vi "Attocube Main.vi"() -> ()   [LabVIEW 2019]
panel:
  out "last move time":timestamp
  out "axis 1:\nCurrent position [µm/°/m°] 2":dbl(knob) scale=65.0..270.0 scale format="%#_3p"
  out "axis 1:\nCurrent position (°)":dbl format="%.4f"
  in  "set static amplitude\nwhen moving":bool
  in  "static amplitude (mV)":dbl=2.0 min=0.001 max=2.0 format="%#_13g"
  in  "both axes: Output":bool caption="both axes:\nOutput"
  in  "axis 2:\nStop moving":bool
  in  "axis 1:\nStop moving":bool
  in  "Remote mode":bool
  in  "axis 2:\nstop detection":bool
  in  "axis 1:\nstop detection":bool
  in  "axis 2:\nOutput":bool
  in  "axis 1:\ncontrol mode":enum16{"speed", "amplitude", "step size"}(ring)=enum."amplitude"
  in  "axis 2:\ncontrol mode":enum16{"speed", "amplitude", "step size"}(ring)=enum."amplitude"
  in  "axis 1:\nOutput":bool
  out "axis 2:\nStepWidth":i32=38 format="%.0fnm"
  out "axis 1:\nStepWidth":i32 format="%.0fnm"
  out "axis 2:\nspeed (°/s)":i32=31
  out "axis 1:\nspeed (°/s)":i32
  out "axis 2:\nCapacitance":i32=2486 format="%.0fnF"
  out "axis 1:\nCapacitance":i32=2534 format="%.0fnF"
  in  "axis 2:\ncap. measure":bool
  in  "axis 1:\ncap. measure":bool
  out "axis 2:\nCurrent position [µm/°/m°] 2":dbl(knob) scale=5.0..320.0
  in  "axis 2:\nFrequency [Hz]":i32=800 min=0 max=20000 format="%.0fHz"
  in  "axis 1:\nFrequency [Hz]":i32=800 min=0 max=20000 format="%.0fHz"
  in  "axis 2:\nDCLevel [V]":dbl min=0.0 max=140.0 step=0.001 format="%.3f"
  in  "axis 1:\nDCLevel [V]":dbl min=0.0 max=140.0 step=0.001 format="%.3f"
  in  "axis 2:\nAmplitude [V]":dbl=35.0 min=0.0 max=150.0 format="%.3gV"
  in  "axis 1:\nAmplitude [V]":dbl=40.0 min=0.0 max=150.0 format="%.3gV"
  in  "axis 2:\ncontinuous back":bool
  in  "axis 2:\ncontinuous fwd":bool
  in  "axis 1:\ncontinuous back":bool
  in  "axis 1:\ncontinuous fwd":bool
  in  "axis 2:\nsingle step fwd":bool
  in  "axis 2:\nsingle step back":bool
  in  "axis 1:\nsingle step back":bool
  in  "axis 1:\nsingle step fwd":bool
  in  "axis 2:\nsp position °":dbl=78.5 min=5.0 max=320.0 format="%.4g"
  in  "axis 2:\nsp rot count":i32
  in  "axis 1:\nsp rot count":i32
  in  "axis 1:\nsp position °":dbl=167.0 min=65.0 max=270.0 format="%.4g"
  in  "axis 2:\nAbsolute":bool
  in  "axis 2:\nRelative":bool
  in  "axis 1:\nRelative":bool
  in  "axis 1:\nAbsolute":bool
  in  "axis 1: \nTarget GND":bool
  in  "axis 1:\nSingle Circle Mode":bool
  in  "axis 2:\nSingle Circle Mode":bool
  in  "axis 2: \nTarget GND":bool
  out "axis 2:\npositioner status":T1
  out "axis 2:\nCurrent position (°)":dbl format="%.4f"
  out "axis 2:\nrot. count":i32
  out "axis 1:\npositioner status":T1
  out "axis 1:\nrot. count":i32
  out "handle":i32=5
  in  "OK":bool
  # "Axis 1: large axis"
  # "Axis 2: small axis"
  # "Notes: \n\n***Switch controller to ground (output=false) before connecting the rotator and while cooling down/warming up***\n\nAxis 1 (large axis): Position is limited by physical stops to angles from 65° to 270°\n\nAxis 2 (small axis): Encoded positions are limited to angles from 5° to 320°, not physically limited to one rotation.  Keep single circle mode OFF to limit the rotation count to zero and protect the wiring from over-rotating.\n\nStatic Amplitude: Sets the voltage applied to the resitive readout system.  Range: 0.001 V to 2V.  Higher voltages enhace the sensitivity but lower voltages minimize heat dissipation for low temperature applications.\n\nAbsolute: positioner travels from its current position to      the target position.\n\nTarget Ground: positioner will be grounded when the target position is reached.\n\nSingle circle mode: If OFF absolute and relative positioning are only allowed up to a full circle, keeps rot count at zero.\n\nOutput: When checked, the repective axis output is enabled.  Deactivating sets the axis to GND\n\nControl mode: \n     amplitude: individual steps of the piezo are definied by        the amplitude.  Driven in open-loop mode, travel speed and step width may vary\n     speed: feedback enables a constant travel speed by closed-loop control of the amplitude and frequency.  Speed is set by adjusting the amplitude and/or frequency values.\n     step width: Step size in controlled to a constant value.  Amplitude is closed-loop controlled.  Step width is set by adjusting the amplitude"
  # "Automatic Positioning"
  # "Automatic Positioning"
  # "Manual Positioning"
  # "Manual Positioning"
  # "Move Single Step"
  # "Move Single Step"
  # "Move Continuous"
  # "Move Continuous"
  # "Capacitance Measurement"
  # "Capacitance Measurement"
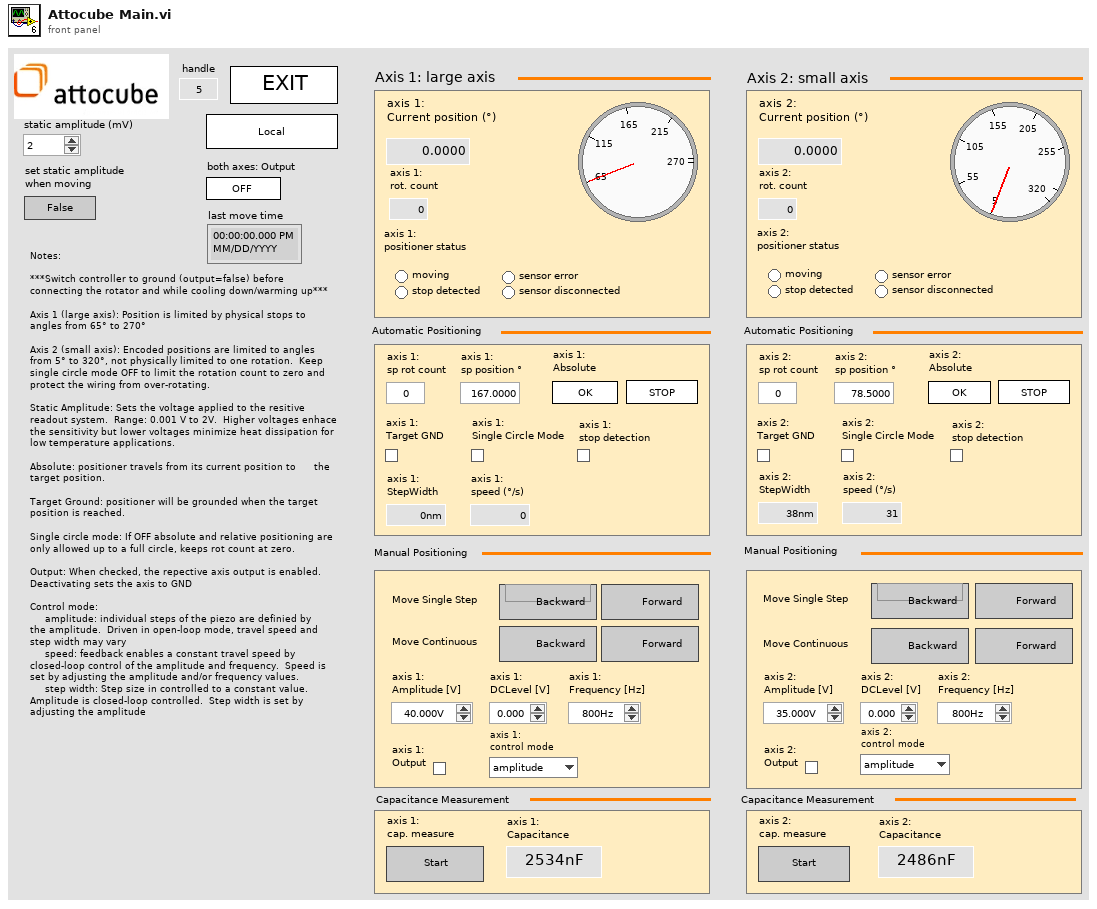
[diagram p1: front panel]
types:
  T1 = cluster{"moving":bool, "stop detected":bool, "sensor error":bool, "sensor disconnected":bool}
  T2 = enum32{"invalid app kind", "Development System", "Run Time System", "Student Edition", "Embedded LabVIEW", "Evaluation", "Custom"}
  T3 = enum32{"Invalid", "Standard", "Closed", "Hidden", "Minimized", "Maximized"}
  T4 = cluster{"axis 1: Absolute":bool, "axis 2: Absolute":bool, "axis 1: Stop moving":bool, "axis 2: Stop moving":bool, "axis 1: Output":bool, "axis 2: Output":bool, "set static amplitude\nwhen moving":bool}
  T5 = cluster{"axis 1: Current position (°)":dbl, "axis 2: Current position (°)":dbl, "axis 1: rot. count":dbl, "axis 2: rot. count":dbl, "axis 1: StepWidth":dbl, "axis 2: StepWidth":dbl, "axis 1: speed (°/s)":dbl, "axis 2: speed (°/s)":dbl, "axis 1: positioner status":cluster{"moving":bool, "stop detected":bool, "sensor error":bool, "sensor disconnected":bool}, "axis 2: positioner status":cluster{"moving":bool, "stop detected":bool, "sensor error":bool, "sensor disconnected":bool}}
  T6 = cluster{"axis 1: Amplitude [V]":dbl, "axis 2: Amplitude [V]":dbl, "axis 1: DCLevel [V]":dbl, "axis 2: DCLevel [V]":dbl, "axis 1: Frequency [Hz]":dbl, "axis 2: Frequency [Hz]":dbl, "axis 1: sp position °":dbl, "axis 2: sp position °":dbl, "axis 1: sp rot count":dbl, "axis 2: sp rot count":dbl}
  T7 = cluster{"error ":bool, "error number":i32, "error code":string}
  T8 = cluster{"Core":cluster{"Current VI Reference":refnum<vi>, "Close Panel on Exit?":bool}, "handle":i32}
  T9 = cluster{"Current VI Reference":refnum<vi>, "Close Panel on Exit?":bool}
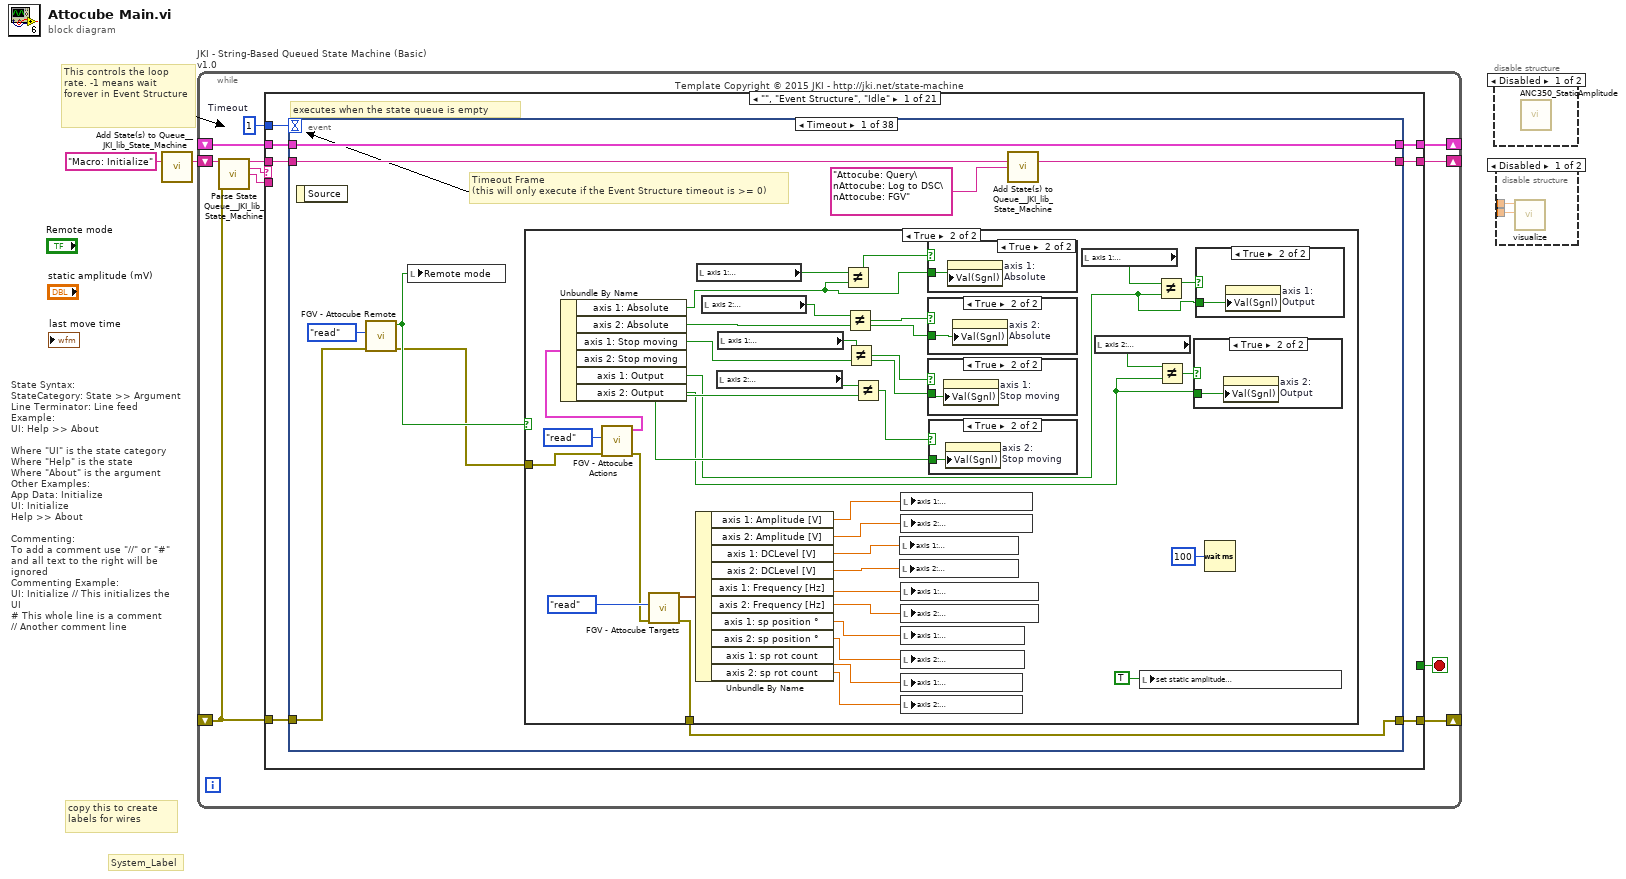
[diagram p0: block diagram]
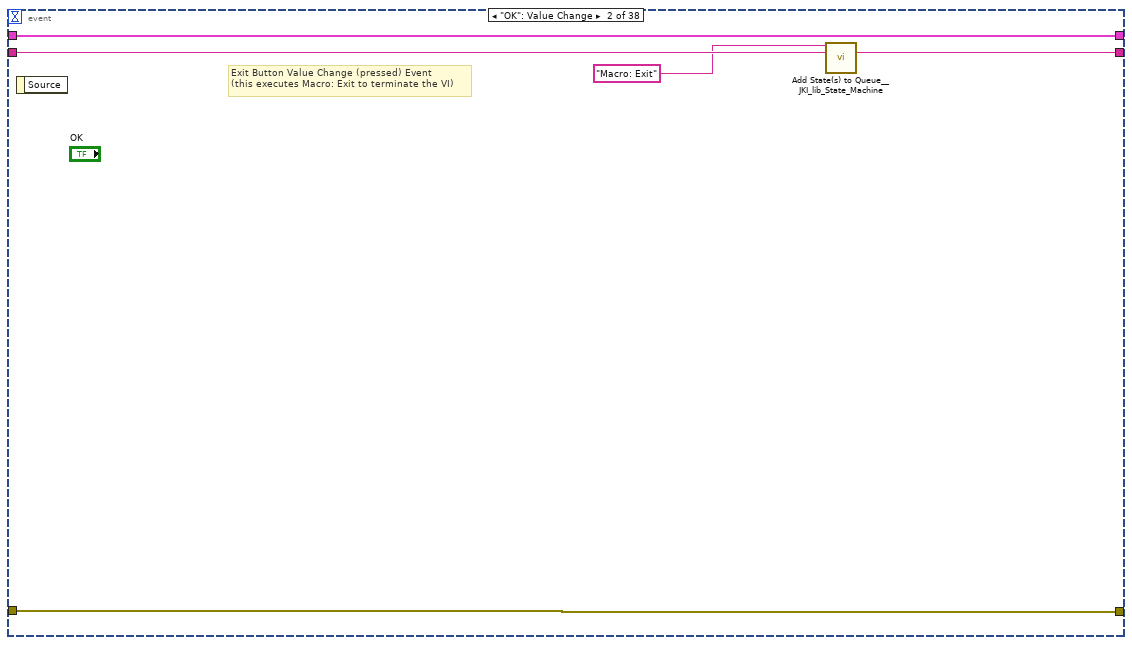
[diagram p11: hidden frame]
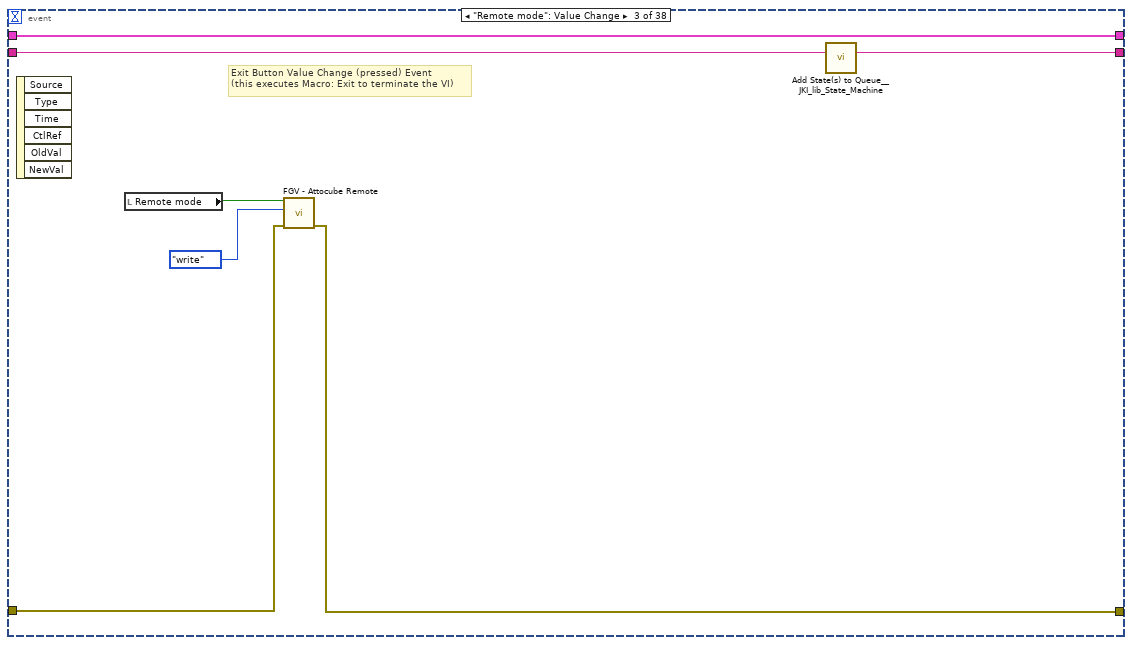
[diagram p12: hidden frame]
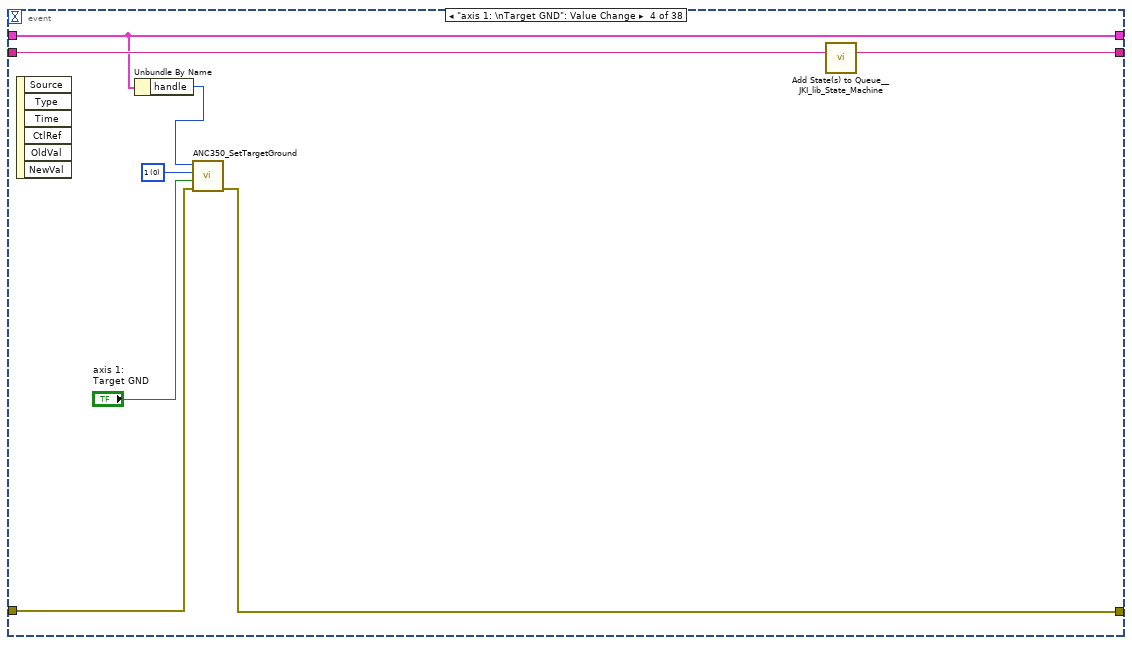
[diagram p13: hidden frame]
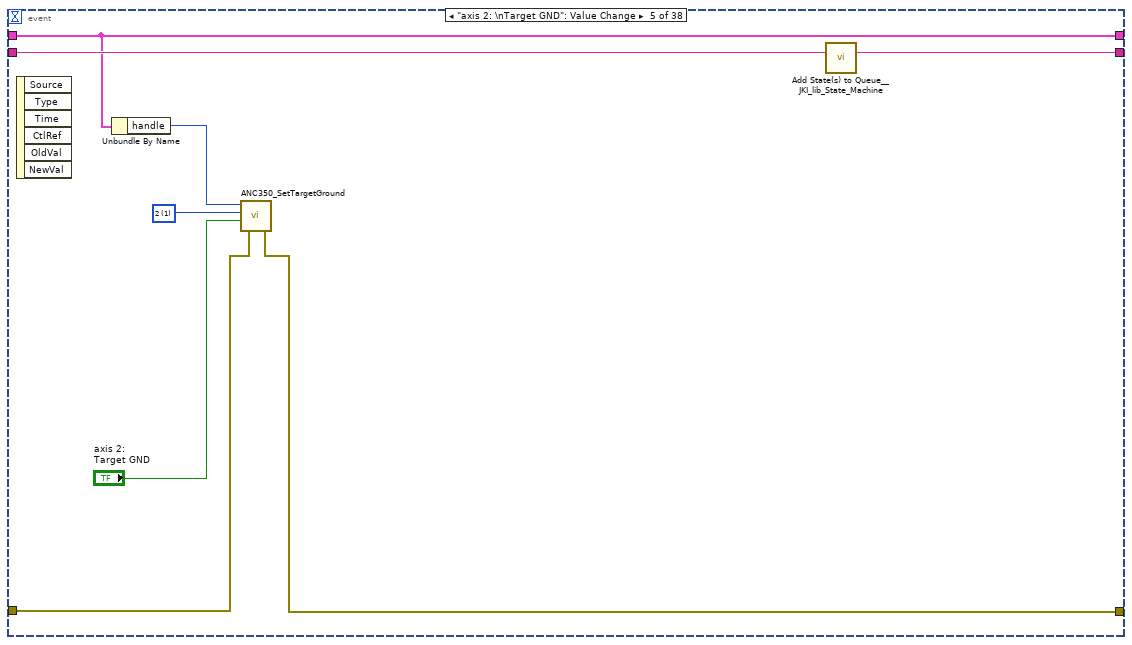
[diagram p14: hidden frame]
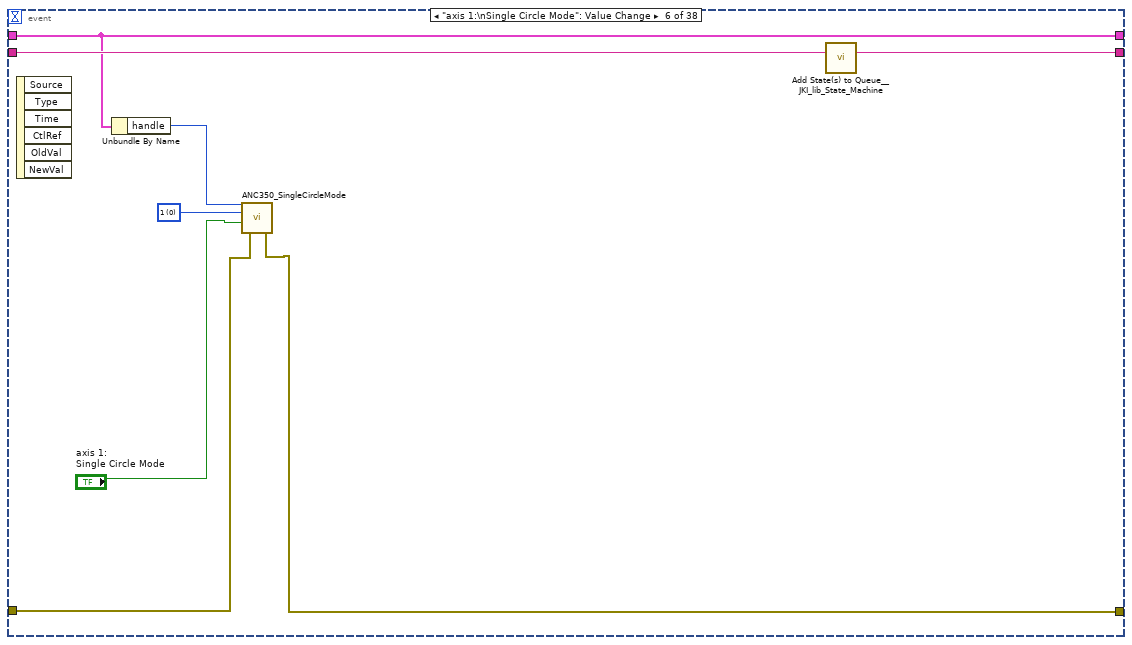
[diagram p15: hidden frame]
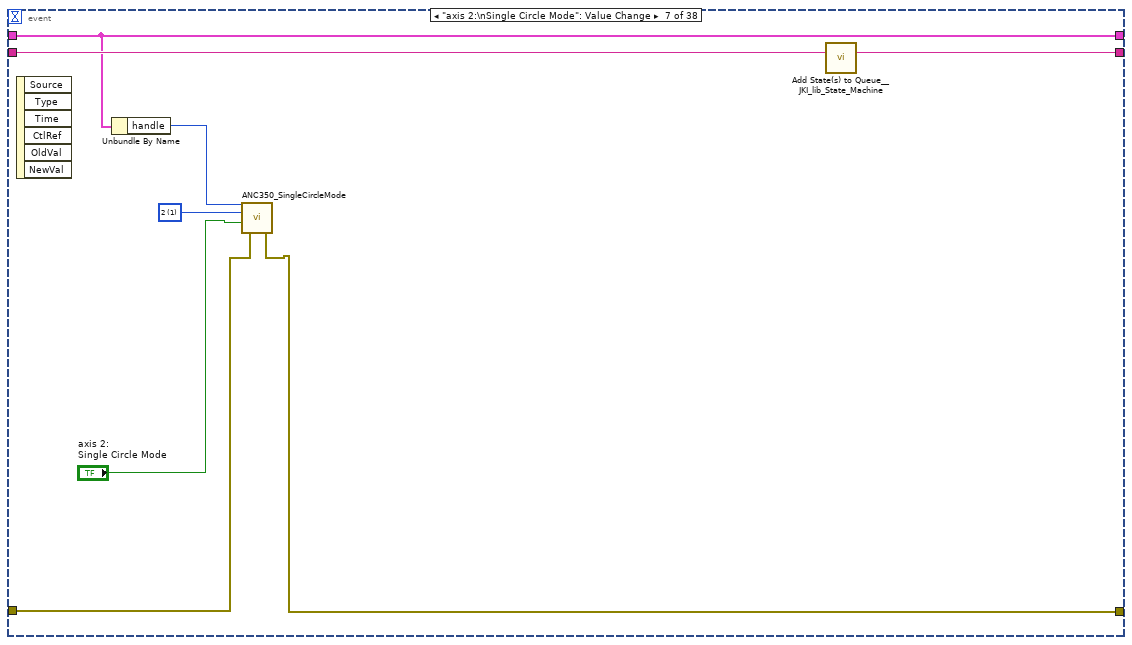
[diagram p16: hidden frame]
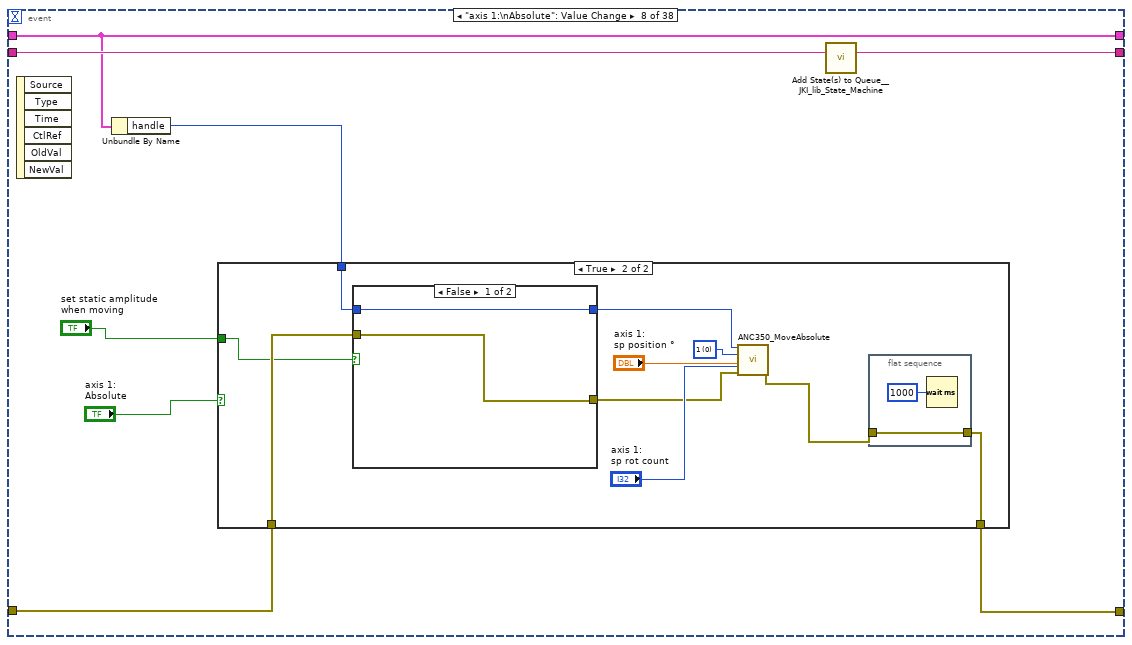
[diagram p17: hidden frame]
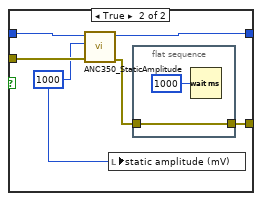
[diagram p19: hidden frame]
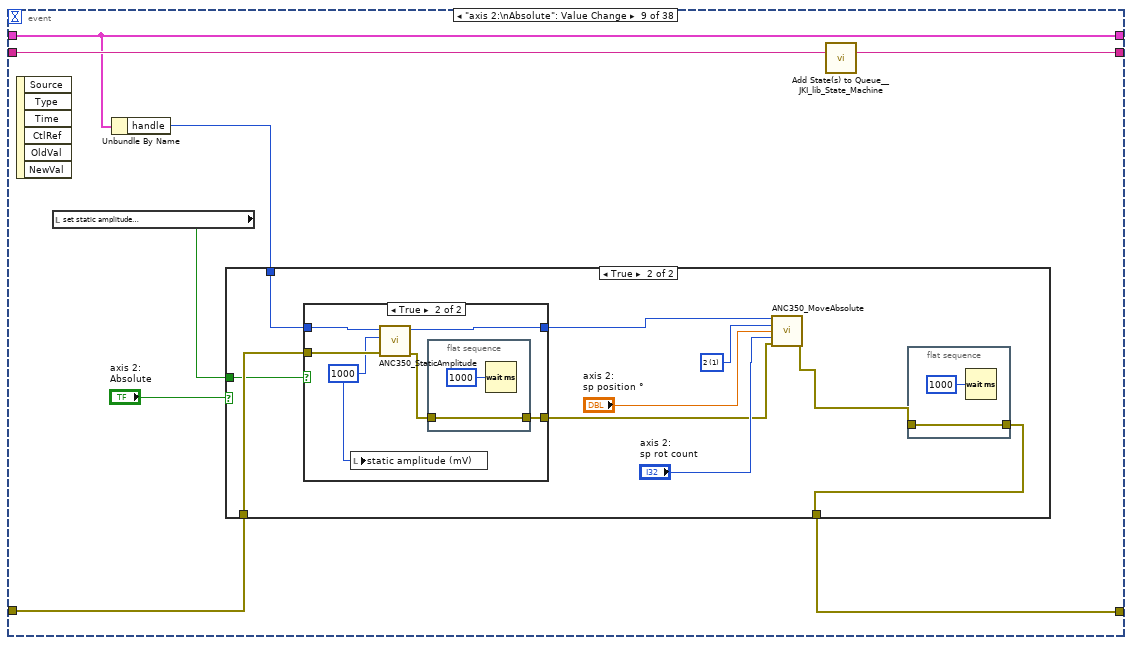
[diagram p20: hidden frame]
diagram:
  # "State Syntax:\nStateCategory: State >> Argument\nLine Terminator: Line feed\nExample:\nUI: Help >> About\n\nWhere \"UI\" is the state category\nWhere \"Help\" is the state\nWhere \"About\" is the argument\nOther Examples:\nApp Data: Initialize\nUI: Initialize\nHelp >> About\n\nCommenting:\nTo add a comment use \"//\" or \"#\" and all text to the right will be ignored\nCommenting Example:\nUI: Initialize // This initializes the UI\n# This whole line is a comment\n// Another comment line"
  # "copy this to create labels for wires"
  # "This controls the loop rate. -1 means wait forever in Event Structure"
  # "System_Label"
  n1 = call <vilib>:"Add State(s) to Queue__JKI_lib_State_Machine.vi"("State(s) in (\"\")"="Macro: Initialize") -> ("States Out"=w2:string)  [unwired: 14 in]
  n2 = while "JKI - String-Based Queued State Machine (Basic) v1.0" {
    shift-right: [w7] -> _
    shift-left: _ -> [w6]
    shift-right: [w3] -> _
    shift-left: _ -> [w4]
    shift-right: [w9] -> _
    shift-left: w2 -> [w10]
    stop <- w8 stop-if-true
    w5 = 1  # Timeout
    # "Template Copyright © 2015 JKI - http://jki.net/state-machine"
    n3 = call <vilib>:"Parse State Queue__JKI_lib_State_Machine.vi"("State Queue"=w10, "Error In (no error)"=w4) -> ("Remaining States"=w12:string, "Current State"=w13:string, "Arguments"=w11:string)  [unwired: 11 in]
    n4 = case shown="\"\", \"Event Structure\", \"Idle\"" w13 {
      selector: w13 -> [_ _ w504 _ _ _ _ _ _ _ _ _ _ _ _ _ _ _ _ _ _]
      tunnel: w12 -> [w20 w503 w508 w526 w532 w537 w541 w547 w553 w557 w568 w579 w590 w616 w621 w647 w651 w666 w736 w797 w850]
      tunnel: w11 -> [_ _ _ _ _ _ _ _ _ _ _ w574 w584 _ _ _ _ _ _ _ _]
      tunnel: w6 -> [w18 w500 w506 w517 w529 w535 w538 _ w548 w554 w566 w577 w586 w613 w618 w645 w648 w664 w734 w795 w848]
      tunnel: w4 -> [w16 w501 w509 w523 w528 w534 w539 w544 w550 w555 w565 w576 w588 w614 w619 w635 w649 _ w733 w750 w815]
      tunnel: [w19 w502 w507 w525 w531 w536 w540 w546 w552 w556 w567 w578 w589 w615 w620 w646 w650 w665 w735 w796 w849] -> w9
      tunnel: [_ _ _ _ _ TRUE _ _ _ _ _ _ _ _ _ _ _ _ _ _ _] -> w8
      tunnel: [w15 w500 w506 w524 w529 w535 w538 w545 w548 w554 w566 w577 w586 w613 w618 w645 w648 w663 w734 w795 w848] -> w7
      tunnel: w5 -> [w14 _ _ _ _ _ _ _ _ _ _ _ _ _ _ _ _ _ _ _ _]
      tunnel: [w17 w501 w510 w523 errorcluster {"status"=FALSE, "code"=0, "source"=""} ("error out") w534 w539 w544 w549 w555 w565 w575 w587 w614 w619 w638 w649 w653 w683 w750 w823] -> w3
      frame "", "Event Structure", "Idle" {
        # "executes when the state queue is empty"
        n5 = event shown="[0] Timeout" {
          selector: _ -> [_ _ _ _ _ _ _ _ _ _ _ _ _ _ _ _ _ _ _ _ _ _ _ _ _ _ _ _ _ _ _ _ _ _ _ _ _ _]
          dyn-events: _ -> [_ _ _ _ _ _ _ _ _ _ _ _ _ _ _ _ _ _ _ _ _ _ _ _ _ _ _ _ _ _ _ _ _ _ _ _ _ _]
          timeout: w14 -> [_ _ _ _ _ _ _ _ _ _ _ _ _ _ _ _ _ _ _ _ _ _ _ _ _ _ _ _ _ _ _ _ _ _ _ _ _ _]
          tunnel: w20 -> [w29 w78 w85 w93 w101 w109 w117 w125 w156 w186 w200 w214 w227 w240 w253 w266 w282 w298 w314 w331 w339 w347 w355 w363 w371 w379 w393 w407 w415 w423 w432 w441 w449 w457 w470 w479 w488 w499]
          tunnel: [w28 w77 w84 w92 w100 w108 w116 w124 w155 w185 w199 w213 w226 w239 w252 w265 w281 w297 w313 w330 w338 w346 w354 w362 w370 w378 w392 w406 w414 w422 w431 w440 w448 w456 w469 w478 w487 w498] -> w19
          tunnel: w18 -> [w27 w75 w83 w91 w99 w107 w115 w123 w154 w184 w198 w212 w225 w238 w251 w264 w280 w296 w312 w329 w337 w345 w353 w361 w369 w377 w391 w405 w413 w421 w430 w439 w447 w455 w468 w477 w486 w496]
          tunnel: [w23 w76 w79 w86 w96 w102 w112 w118 w151 w181 w195 w209 w222 w235 w248 w261 w277 w293 w309 w324 w333 w340 w349 w356 w365 w373 w387 w401 w409 w418 w427 w435 w443 w451 w464 w476 w483 w497] -> w17
          tunnel: w16 -> [w22 w76 w80 w87 w97 w103 w113 w121 w152 w182 w196 w210 w223 w236 w249 w262 w278 w294 w310 w325 w334 w341 w350 w357 w366 w374 w388 w402 w410 w419 w428 w436 w444 w452 w465 w476 w484 w497]
          tunnel: [w27 w75 w83 w91 w99 w107 w115 w123 w154 w184 w198 w212 w225 w238 w251 w264 w280 w296 w312 w329 w337 w345 w353 w361 w369 w377 w391 w405 w413 w421 w430 w439 w447 w455 w468 w477 w486 w496] -> w15
          event Timeout {
            # "Timeout Frame\n(this will only execute if the Event Structure timeout is >= 0)"
            n6 = event-data() -> ()  [unwired: 1 in, 1 out]
            n7 = call "FGV - Attocube Remote.vi"("error in"=w22, "Function"=enum16{"write", "read"}."read") -> ("error out"=w21:errorcluster, "Attocube Remote"=w24:bool)  [unwired: 4 in]
            n8 = local write "Remote mode"(w24) -> ()
            n9 = case shown="True" w24 {
              tunnel: w21 -> [w30 w34]
              tunnel: [w30 w32] -> w23
              frame False {
              }
              frame True {
                n10 = call "FGV - Attocube Actions.vi"("error in"=w34, "Function"=enum16{"write", "read"}."read") -> ("error out"=w33:errorcluster, "Actions OUT"=w66:T4)  [unwired: 4 in]
                n11 = Unbundle By Name(w66) -> ("axis 1: Absolute"=w60:bool, "axis 2: Absolute"=w59:bool, "axis 1: Stop moving"=w55:bool, "axis 2: Stop moving"=w54:bool, "axis 1: Output"=w39:bool, "axis 2: Output"=w36:bool)
                n12 = call "FGV - Attocube Targets.vi"("error in"=w33, "Function"=enum16{"write", "read"}."read") -> ("error out"=w32:errorcluster, "Targets Out"=w52:T6)  [unwired: 4 in]
                n13 = Unbundle By Name(w52) -> ("axis 1: Amplitude [V]"=w51:dbl, "axis 2: Amplitude [V]"=w50:dbl, "axis 1: DCLevel [V]"=w49:dbl, "axis 2: DCLevel [V]"=w48:dbl, "axis 1: Frequency [Hz]"=w47:dbl, "axis 2: Frequency [Hz]"=w46:dbl, "axis 1: sp position °"=w31:dbl, "axis 2: sp position °"=w45:dbl, "axis 1: sp rot count"=w44:dbl, "axis 2: sp rot count"=w43:dbl)
                n14 = local read "axis 1:\nAbsolute"() -> (w65:bool)
                n15 = local read "axis 2:\nAbsolute"() -> (w64:bool)
                n16 = local read "axis 2:\nStop moving"() -> (w62:bool)
                n17 = local read "axis 1:\nStop moving"() -> (w63:bool)
                n18 = Not Equal?(x=w65, y=w60) -> (x != y?=w61:bool)
                n19 = Not Equal?(x=w64, y=w59) -> (x != y?=w58:bool)
                n20 = Not Equal?(x=w63, y=w55) -> (x != y?=w57:bool)
                n21 = Not Equal?(x=w62, y=w54) -> (x != y?=w56:bool)
                n22 = local write "axis 1:\nDCLevel [V]"(w49) -> ()
                n23 = local write "axis 2:\nDCLevel [V]"(w48) -> ()
                n24 = local write "axis 1:\nAmplitude [V]"(w51) -> ()
                n25 = local write "axis 2:\nAmplitude [V]"(w50) -> ()
                n26 = local write "axis 1:\nFrequency [Hz]"(w47) -> ()
                n27 = local write "axis 2:\nFrequency [Hz]"(w46) -> ()
                n28 = local write "axis 1:\nsp position °"(w31) -> ()
                n29 = local write "axis 2:\nsp position °"(w45) -> ()
                n30 = local write "axis 1:\nsp rot count"(w44) -> ()
                n31 = local write "axis 2:\nsp rot count"(w43) -> ()
                n32 = case shown="True" w61 {
                  tunnel: w60 -> [_ w73]
                  frame False {
                  }
                  frame True {
                    n33 = property on="axis 1:\nAbsolute" class="Bool (strict)"("Val(Sgnl)"=w73) -> ()  [unwired: 2 in, 2 out]
                  }
                }
                n34 = case shown="True" w58 {
                  tunnel: w59 -> [_ w72]
                  frame False {
                  }
                  frame True {
                    n35 = property on="axis 2:\nAbsolute" class="Bool (strict)"("Val(Sgnl)"=w72) -> ()  [unwired: 2 in, 2 out]
                  }
                }
                n36 = case shown="True" w57 {
                  tunnel: w55 -> [_ w71]
                  frame False {
                  }
                  frame True {
                    n37 = property on="axis 1:\nStop moving" class="Bool (strict)"("Val(Sgnl)"=w71) -> ()  [unwired: 2 in, 2 out]
                  }
                }
                n38 = case shown="True" w56 {
                  tunnel: w54 -> [_ w70]
                  frame False {
                  }
                  frame True {
                    n39 = property on="axis 2:\nStop moving" class="Bool (strict)"("Val(Sgnl)"=w70) -> ()  [unwired: 2 in, 2 out]
                  }
                }
                n40 = local read "axis 1:\nOutput"() -> (w40:bool)
                n41 = local read "axis 2:\nOutput"() -> (w37:bool)
                n42 = local write "set static amplitude\nwhen moving"(TRUE) -> ()
                n43 = Not Equal?(x=w40, y=w39) -> (x != y?=w41:bool)
                n44 = Not Equal?(x=w37, y=w36) -> (x != y?=w38:bool)
                n45 = case shown="True" w38 {
                  tunnel: w36 -> [_ w68]
                  frame False {
                  }
                  frame True {
                    n46 = property on="axis 2:\nOutput" class="Bool (strict)"("Val(Sgnl)"=w68) -> ()  [unwired: 2 in, 2 out]
                  }
                }
                n47 = case shown="True" w41 {
                  tunnel: w39 -> [_ w69]
                  frame False {
                  }
                  frame True {
                    n48 = property on="axis 1:\nOutput" class="Bool (strict)"("Val(Sgnl)"=w69) -> ()  [unwired: 2 in, 2 out]
                  }
                }
                n49 = Wait (ms)(milliseconds to wait=u32 100) -> ()  [unwired: 1 out]
              }
            }
            n50 = call <vilib>:"Add State(s) to Queue__JKI_lib_State_Machine.vi"("State(s) in (\"\")"=w29, "State(s) at Back (\"\")"="Attocube: Query\nAttocube: Log to DSC\nAttocube: FGV" ("State(s) at Back (\"\")")) -> ("States Out"=w28:string)  [unwired: 13 in]
          }
          event "OK": Value Change {
            # "Exit Button Value Change (pressed) Event\n(this executes Macro: Exit to terminate the VI)"
            n51 = event-data() -> ()  [unwired: 1 in, 1 out]
            n52 = call <vilib>:"Add State(s) to Queue__JKI_lib_State_Machine.vi"("State(s) in Front (\"\")"="Macro: Exit", "State(s) in (\"\")"=w78) -> ("States Out"=w77:string)  [unwired: 13 in]
          }
          event "Remote mode": Value Change {
            # "Exit Button Value Change (pressed) Event\n(this executes Macro: Exit to terminate the VI)"
            n53 = event-data() -> ()  [unwired: 1 in, 6 out]
            n54 = local read "Remote mode"() -> (w82:bool)
            n55 = call "FGV - Attocube Remote.vi"("error in"=w80, "Function"=enum16{"write", "read"}."write", "Attocube Remote"=w82) -> ("error out"=w79:errorcluster)  [unwired: 3 in, 1 out]
            n56 = call <vilib>:"Add State(s) to Queue__JKI_lib_State_Machine.vi"("State(s) in (\"\")"=w85) -> ("States Out"=w84:string)  [unwired: 14 in]
          }
          event "axis 1: \nTarget GND": Value Change {
            w89 = u8 0 items=["1", "2", "3", "4", "5", "6", "7", "8", "9"] ("axis no")
            n57 = event-data() -> ()  [unwired: 1 in, 6 out]
            n58 = Unbundle By Name(w91) -> ("handle"=w90:i32)
            n59 = call "ANC350_SetTargetGround.vi"("error in"=w87, "PositionerAcIn"="axis 1: \nTarget GND", "axis no"=w89, "device handle"=w90) -> ("error out"=w86:T7)  [unwired: 2 in, 1 out]
            n60 = call <vilib>:"Add State(s) to Queue__JKI_lib_State_Machine.vi"("State(s) in (\"\")"=w93) -> ("States Out"=w92:string)  [unwired: 14 in]
          }
          event "axis 2: \nTarget GND": Value Change {
            w95 = u8 1 items=["1", "2", "3", "4", "5", "6", "7", "8", "9"] ("axis no")
            n61 = event-data() -> ()  [unwired: 1 in, 6 out]
            n62 = Unbundle By Name(w99) -> ("handle"=w98:i32)
            n63 = call "ANC350_SetTargetGround.vi"("error in"=w97, "PositionerAcIn"="axis 2: \nTarget GND", "axis no"=w95, "device handle"=w98) -> ("error out"=w96:T7)  [unwired: 2 in, 1 out]
            n64 = call <vilib>:"Add State(s) to Queue__JKI_lib_State_Machine.vi"("State(s) in (\"\")"=w101) -> ("States Out"=w100:string)  [unwired: 14 in]
          }
          event "axis 1:\nSingle Circle Mode": Value Change {
            w105 = u8 0 items=["1", "2", "3", "4", "5", "6", "7", "8", "9"] ("axis no")
            n65 = event-data() -> ()  [unwired: 1 in, 6 out]
            n66 = Unbundle By Name(w107) -> ("handle"=w106:i32)
            n67 = call "ANC350_SingleCircleMode.vi"("error in"=w103, "enable"="axis 1:\nSingle Circle Mode", "axis no"=w105, "device handle"=w106) -> ("error out"=w102:T7)  [unwired: 2 in, 1 out]
            n68 = call <vilib>:"Add State(s) to Queue__JKI_lib_State_Machine.vi"("State(s) in (\"\")"=w109) -> ("States Out"=w108:string)  [unwired: 14 in]
          }
          event "axis 2:\nSingle Circle Mode": Value Change {
            w110 = u8 1 items=["1", "2", "3", "4", "5", "6", "7", "8", "9"] ("axis no")
            n69 = event-data() -> ()  [unwired: 1 in, 6 out]
            n70 = Unbundle By Name(w115) -> ("handle"=w114:i32)
            n71 = call "ANC350_SingleCircleMode.vi"("error in"=w113, "enable"="axis 2:\nSingle Circle Mode", "axis no"=w110, "device handle"=w114) -> ("error out"=w112:T7)  [unwired: 2 in, 1 out]
            n72 = call <vilib>:"Add State(s) to Queue__JKI_lib_State_Machine.vi"("State(s) in (\"\")"=w117) -> ("States Out"=w116:string)  [unwired: 14 in]
          }
          event "axis 1:\nAbsolute": Value Change {
            n73 = event-data() -> ()  [unwired: 1 in, 6 out]
            n74 = Unbundle By Name(w123) -> ("handle"=w122:i32)
            n75 = case shown="True" "axis 1:\nAbsolute" {
              tunnel: w122 -> [_ w133]
              tunnel: w121 -> [w126 w131]
              tunnel: "set static amplitude\nwhen moving" -> [_ w129]
              tunnel: [w126 w127] -> w118
              frame False {
              }
              frame True {
                w136 = u8 0 items=["1", "2", "3", "4", "5", "6", "7", "8", "9"] ("axis no")
                n76 = case shown="False" w129 {
                  tunnel: w133 -> [w140 w146]
                  tunnel: [w140 w145] -> w132
                  tunnel: w131 -> [w139 w144]
                  tunnel: [w139 w142] -> w130
                  frame False {
                  }
                  frame True {
                    w141 = 1000 ("static amplitude")
                    n77 = call "ANC350_StaticAmplitude.vi"("error in"=w144, "static amplitude"=w141, "device handle"=w146) -> ("error out"=w143:T7, "device handle Out"=w145:i32)  [unwired: 3 in]
                    n78 = local write "static amplitude (mV)"(w141) -> ()
                    n79 = flat-sequence {
                      tunnel: [w148] -> w142
                      tunnel: w143 -> [w148]
                      frame #0 {
                        n80 = Wait (ms)(milliseconds to wait=u32 1000) -> ()  [unwired: 1 out]
                      }
                    }
                  }
                }
                n81 = call "ANC350_MoveAbsolute.vi"("device handle"=w132, "axis no"=w136, "absoluteposition [µm/°/m°]"="axis 1:\nsp position °", "rot count"="axis 1:\nsp rot count", "error in"=w130) -> ("error out"=w128:T7)  [unwired: 9 in, 1 out]
                n82 = flat-sequence {
                  tunnel: [w138] -> w127
                  tunnel: w128 -> [w138]
                  frame #0 {
                    n83 = Wait (ms)(milliseconds to wait=u32 1000) -> ()  [unwired: 1 out]
                  }
                }
              }
            }
            n84 = call <vilib>:"Add State(s) to Queue__JKI_lib_State_Machine.vi"("State(s) in (\"\")"=w125) -> ("States Out"=w124:string)  [unwired: 14 in]
          }
          event "axis 2:\nAbsolute": Value Change {
            n85 = event-data() -> ()  [unwired: 1 in, 6 out]
            n86 = local read "set static amplitude\nwhen moving"() -> (w149:bool)
            n87 = Unbundle By Name(w154) -> ("handle"=w153:i32)
            n88 = case shown="True" "axis 2:\nAbsolute" {
              tunnel: w153 -> [_ w164]
              tunnel: w152 -> [w157 w162]
              tunnel: [w157 w158] -> w151
              tunnel: w149 -> [_ w160]
              frame False {
              }
              frame True {
                w167 = u8 1 items=["1", "2", "3", "4", "5", "6", "7", "8", "9"] ("axis no")
                n89 = case shown="True" w160 {
                  tunnel: w164 -> [w171 w177]
                  tunnel: [w171 w176] -> w163
                  tunnel: w162 -> [w170 w175]
                  tunnel: [w170 w173] -> w161
                  frame False {
                  }
                  frame True {
                    w172 = 1000 ("static amplitude")
                    n90 = local write "static amplitude (mV)"(w172) -> ()
                    n91 = call "ANC350_StaticAmplitude.vi"("error in"=w175, "static amplitude"=w172, "device handle"=w177) -> ("error out"=w174:T7, "device handle Out"=w176:i32)  [unwired: 3 in]
                    n92 = flat-sequence {
                      tunnel: [w179] -> w173
                      tunnel: w174 -> [w179]
                      frame #0 {
                        n93 = Wait (ms)(milliseconds to wait=u32 1000) -> ()  [unwired: 1 out]
                      }
                    }
                  }
                }
                n94 = call "ANC350_MoveAbsolute.vi"("device handle"=w163, "axis no"=w167, "absoluteposition [µm/°/m°]"="axis 2:\nsp position °", "rot count"="axis 2:\nsp rot count", "error in"=w161) -> ("error out"=w159:T7)  [unwired: 9 in, 1 out]
                n95 = flat-sequence {
                  tunnel: [w169] -> w158
                  tunnel: w159 -> [w169]
                  frame #0 {
                    n96 = Wait (ms)(milliseconds to wait=u32 1000) -> ()  [unwired: 1 out]
                  }
                }
              }
            }
            n97 = call <vilib>:"Add State(s) to Queue__JKI_lib_State_Machine.vi"("State(s) in (\"\")"=w156) -> ("States Out"=w155:string)  [unwired: 14 in]
          }
          event "axis 1:\nRelative": Value Change {
            n98 = event-data() -> ()  [unwired: 1 in, 6 out]
            n99 = disable-structure shown="Disabled" {
              frame Disabled {
              }
              frame Enabled {
              }
            }
            n100 = Unbundle By Name(w184) -> ("handle"=w183:i32)
            n101 = case shown="True" FALSE {
              tunnel: w183 -> [_ w193]
              tunnel: w182 -> [w187 w191]
              tunnel: [w187 w188] -> w181
              frame False {
              }
              frame True {
                w192 = u8 0 items=["1", "2", "3", "4", "5", "6", "7", "8", "9"] ("axis no")
                n102 = local read "axis 1:\nsp position °"() -> (w190:dbl)
                n103 = local read "axis 1:\nsp rot count"() -> (w189:i32)
                n104 = call "ANC350_MoveRelative.vi"("device handle"=w193, "axis no"=w192, "distance [µm/°/m°]"=w190, "rot count"=w189, "error in"=w191) -> ("error out"=w188:T7)  [unwired: 9 in, 1 out]
              }
            }
            n105 = call <vilib>:"Add State(s) to Queue__JKI_lib_State_Machine.vi"("State(s) in (\"\")"=w186) -> ("States Out"=w185:string)  [unwired: 14 in]
          }
          event "axis 2:\nRelative": Value Change {
            n106 = event-data() -> ()  [unwired: 1 in, 6 out]
            n107 = disable-structure shown="Disabled" {
              frame Disabled {
              }
              frame Enabled {
              }
            }
            n108 = Unbundle By Name(w198) -> ("handle"=w197:i32)
            n109 = case shown="True" FALSE {
              tunnel: w197 -> [_ w207]
              tunnel: w196 -> [w201 w205]
              tunnel: [w201 w204] -> w195
              frame False {
              }
              frame True {
                w206 = u8 1 items=["1", "2", "3", "4", "5", "6", "7", "8", "9"] ("axis no")
                n110 = local read "axis 2:\nsp position °"() -> (w203:dbl)
                n111 = local read "axis 2:\nsp rot count"() -> (w202:i32)
                n112 = call "ANC350_MoveRelative.vi"("device handle"=w207, "axis no"=w206, "distance [µm/°/m°]"=w203, "rot count"=w202, "error in"=w205) -> ("error out"=w204:T7)  [unwired: 9 in, 1 out]
              }
            }
            n113 = call <vilib>:"Add State(s) to Queue__JKI_lib_State_Machine.vi"("State(s) in (\"\")"=w200) -> ("States Out"=w199:string)  [unwired: 14 in]
          }
          event "axis 1:\nsingle step fwd": Value Change {
            n114 = event-data() -> ()  [unwired: 1 in, 6 out]
            n115 = Unbundle By Name(w212) -> ("handle"=w211:i32)
            n116 = case shown="True" "axis 1:\nsingle step fwd" {
              tunnel: w211 -> [_ w220]
              tunnel: w210 -> [w215 w217]
              tunnel: [w215 w216] -> w209
              frame False {
              }
              frame True {
                w219 = u8 0 items=["1", "2", "3", "4", "5", "6", "7", "8", "9"] ("axis no")
                n117 = call "ANC350_MoveSingleStep.vi"("error in"=w217, "single step direction"=FALSE, "axis no"=w219, "device handle"=w220) -> ("error out"=w216:T7)  [unwired: 2 in, 1 out]
              }
            }
            n118 = call <vilib>:"Add State(s) to Queue__JKI_lib_State_Machine.vi"("State(s) in (\"\")"=w214) -> ("States Out"=w213:string)  [unwired: 14 in]
          }
          event "axis 1:\nsingle step back": Value Change {
            n119 = event-data() -> ()  [unwired: 1 in, 6 out]
            n120 = Unbundle By Name(w225) -> ("handle"=w224:i32)
            n121 = case shown="True" "axis 1:\nsingle step back" {
              tunnel: w224 -> [_ w233]
              tunnel: w223 -> [w228 w230]
              tunnel: [w228 w229] -> w222
              frame False {
              }
              frame True {
                w232 = u8 0 items=["1", "2", "3", "4", "5", "6", "7", "8", "9"] ("axis no")
                n122 = call "ANC350_MoveSingleStep.vi"("error in"=w230, "single step direction"=TRUE, "axis no"=w232, "device handle"=w233) -> ("error out"=w229:T7)  [unwired: 2 in, 1 out]
              }
            }
            n123 = call <vilib>:"Add State(s) to Queue__JKI_lib_State_Machine.vi"("State(s) in (\"\")"=w227) -> ("States Out"=w226:string)  [unwired: 14 in]
          }
          event "axis 2:\nsingle step fwd": Value Change {
            n124 = event-data() -> ()  [unwired: 1 in, 6 out]
            n125 = Unbundle By Name(w238) -> ("handle"=w237:i32)
            n126 = case shown="True" "axis 2:\nsingle step fwd" {
              tunnel: w237 -> [_ w246]
              tunnel: w236 -> [w241 w243]
              tunnel: [w241 w242] -> w235
              frame False {
              }
              frame True {
                w245 = u8 1 items=["1", "2", "3", "4", "5", "6", "7", "8", "9"] ("axis no")
                n127 = call "ANC350_MoveSingleStep.vi"("error in"=w243, "single step direction"=FALSE, "axis no"=w245, "device handle"=w246) -> ("error out"=w242:T7)  [unwired: 2 in, 1 out]
              }
            }
            n128 = call <vilib>:"Add State(s) to Queue__JKI_lib_State_Machine.vi"("State(s) in (\"\")"=w240) -> ("States Out"=w239:string)  [unwired: 14 in]
          }
          event "axis 2:\nsingle step back": Value Change {
            n129 = event-data() -> ()  [unwired: 1 in, 6 out]
            n130 = Unbundle By Name(w251) -> ("handle"=w250:i32)
            n131 = case shown="True" "axis 2:\nsingle step back" {
              tunnel: w250 -> [_ w259]
              tunnel: w249 -> [w254 w256]
              tunnel: [w254 w255] -> w248
              frame False {
              }
              frame True {
                w258 = u8 1 items=["1", "2", "3", "4", "5", "6", "7", "8", "9"] ("axis no")
                n132 = call "ANC350_MoveSingleStep.vi"("error in"=w256, "single step direction"=TRUE, "axis no"=w258, "device handle"=w259) -> ("error out"=w255:T7)  [unwired: 2 in, 1 out]
              }
            }
            n133 = call <vilib>:"Add State(s) to Queue__JKI_lib_State_Machine.vi"("State(s) in (\"\")"=w253) -> ("States Out"=w252:string)  [unwired: 14 in]
          }
          event "axis 1:\ncontinuous fwd": Value Change {
            n134 = event-data() -> ()  [unwired: 1 in, 6 out]
            n135 = Unbundle By Name(w264) -> ("handle"=w263:i32)
            n136 = case shown="True" "axis 1:\ncontinuous fwd" {
              tunnel: w263 -> [w270 w275]
              tunnel: w262 -> [w269 w273]
              tunnel: [w268 w272] -> w261
              frame False {
                w267 = u8 0 items=["1", "2", "3", "4", "5", "6", "7", "8", "9"] ("axis no")
                n137 = call "ANC350_StopMoving.vi"("error in"=w269, "axis no"=w267, "device handle"=w270) -> ("error out"=w268:T7)  [unwired: 3 in, 1 out]
              }
              frame True {
                w274 = u8 0 items=["1", "2", "3", "4", "5", "6", "7", "8", "9"] ("axis no")
                n138 = call "ANC350_MoveContinuous.vi"("error in"=w273, "step direction"=FALSE ("single step direction"), "axis no"=w274, "device handle"=w275) -> ("error out"=w272:T7)  [unwired: 2 in, 1 out]
              }
            }
            n139 = call <vilib>:"Add State(s) to Queue__JKI_lib_State_Machine.vi"("State(s) in (\"\")"=w266) -> ("States Out"=w265:string)  [unwired: 14 in]
          }
          event "axis 1:\ncontinuous back": Value Change {
            n140 = event-data() -> ()  [unwired: 1 in, 6 out]
            n141 = Unbundle By Name(w280) -> ("handle"=w279:i32)
            n142 = case shown="True" "axis 1:\ncontinuous back" {
              tunnel: w279 -> [w286 w291]
              tunnel: w278 -> [w285 w289]
              tunnel: [w284 w288] -> w277
              frame False {
                w283 = u8 0 items=["1", "2", "3", "4", "5", "6", "7", "8", "9"] ("axis no")
                n143 = call "ANC350_StopMoving.vi"("error in"=w285, "axis no"=w283, "device handle"=w286) -> ("error out"=w284:T7)  [unwired: 3 in, 1 out]
              }
              frame True {
                w290 = u8 0 items=["1", "2", "3", "4", "5", "6", "7", "8", "9"] ("axis no")
                n144 = call "ANC350_MoveContinuous.vi"("error in"=w289, "step direction"=TRUE ("single step direction"), "axis no"=w290, "device handle"=w291) -> ("error out"=w288:T7)  [unwired: 2 in, 1 out]
              }
            }
            n145 = call <vilib>:"Add State(s) to Queue__JKI_lib_State_Machine.vi"("State(s) in (\"\")"=w282) -> ("States Out"=w281:string)  [unwired: 14 in]
          }
          event "axis 2:\ncontinuous fwd": Value Change {
            n146 = event-data() -> ()  [unwired: 1 in, 6 out]
            n147 = Unbundle By Name(w296) -> ("handle"=w295:i32)
            n148 = case shown="True" "axis 2:\ncontinuous fwd" {
              tunnel: w295 -> [w302 w307]
              tunnel: w294 -> [w301 w305]
              tunnel: [w300 w304] -> w293
              frame False {
                w299 = u8 1 items=["1", "2", "3", "4", "5", "6", "7", "8", "9"] ("axis no")
                n149 = call "ANC350_StopMoving.vi"("error in"=w301, "axis no"=w299, "device handle"=w302) -> ("error out"=w300:T7)  [unwired: 3 in, 1 out]
              }
              frame True {
                w306 = u8 1 items=["1", "2", "3", "4", "5", "6", "7", "8", "9"] ("axis no")
                n150 = call "ANC350_MoveContinuous.vi"("error in"=w305, "step direction"=FALSE ("single step direction"), "axis no"=w306, "device handle"=w307) -> ("error out"=w304:T7)  [unwired: 2 in, 1 out]
              }
            }
            n151 = call <vilib>:"Add State(s) to Queue__JKI_lib_State_Machine.vi"("State(s) in (\"\")"=w298) -> ("States Out"=w297:string)  [unwired: 14 in]
          }
          event "axis 2:\ncontinuous back": Value Change {
            n152 = event-data() -> ()  [unwired: 1 in, 6 out]
            n153 = Unbundle By Name(w312) -> ("handle"=w311:i32)
            n154 = case shown="False" "axis 2:\ncontinuous back" {
              tunnel: w311 -> [w318 w323]
              tunnel: w310 -> [w317 w321]
              tunnel: [w316 w320] -> w309
              frame False {
                w315 = u8 1 items=["1", "2", "3", "4", "5", "6", "7", "8", "9"] ("axis no")
                n155 = call "ANC350_StopMoving.vi"("error in"=w317, "axis no"=w315, "device handle"=w318) -> ("error out"=w316:T7)  [unwired: 3 in, 1 out]
              }
              frame True {
                w322 = u8 1 items=["1", "2", "3", "4", "5", "6", "7", "8", "9"] ("axis no")
                n156 = call "ANC350_MoveContinuous.vi"("error in"=w321, "step direction"=TRUE ("single step direction"), "axis no"=w322, "device handle"=w323) -> ("error out"=w320:T7)  [unwired: 2 in, 1 out]
              }
            }
            n157 = call <vilib>:"Add State(s) to Queue__JKI_lib_State_Machine.vi"("State(s) in (\"\")"=w314) -> ("States Out"=w313:string)  [unwired: 14 in]
          }
          event "axis 1:\nAmplitude [V]": Value Change {
            w327 = u8 0 items=["1", "2", "3", "4", "5", "6", "7", "8", "9"] ("axis no")
            n158 = event-data() -> ()  [unwired: 1 in, 6 out]
            n159 = Unbundle By Name(w329) -> ("handle"=w328:i32)
            n160 = call "ANC350_Amplitude.vi"("error in"=w325, "PositionerAmplitude [V]"="axis 1:\nAmplitude [V]", "axis no"=w327, "device handle"=w328) -> ("error out"=w324:T7)  [unwired: 2 in, 1 out]
            n161 = call <vilib>:"Add State(s) to Queue__JKI_lib_State_Machine.vi"("State(s) in (\"\")"=w331) -> ("States Out"=w330:string)  [unwired: 14 in]
          }
          event "axis 2:\nAmplitude [V]": Value Change {
            w335 = u8 1 items=["1", "2", "3", "4", "5", "6", "7", "8", "9"] ("axis no")
            n162 = event-data() -> ()  [unwired: 1 in, 6 out]
            n163 = Unbundle By Name(w337) -> ("handle"=w336:i32)
            n164 = call "ANC350_Amplitude.vi"("error in"=w334, "PositionerAmplitude [V]"="axis 2:\nAmplitude [V]", "axis no"=w335, "device handle"=w336) -> ("error out"=w333:T7)  [unwired: 2 in, 1 out]
            n165 = call <vilib>:"Add State(s) to Queue__JKI_lib_State_Machine.vi"("State(s) in (\"\")"=w339) -> ("States Out"=w338:string)  [unwired: 14 in]
          }
          event "axis 1:\nDCLevel [V]": Value Change {
            w343 = u8 0 items=["1", "2", "3", "4", "5", "6", "7", "8", "9"] ("axis no")
            n166 = event-data() -> ()  [unwired: 1 in, 6 out]
            n167 = Unbundle By Name(w345) -> ("handle"=w344:i32)
            n168 = call "ANC350_DCLevel.vi"("error in"=w341, "DCLevel [V]"="axis 1:\nDCLevel [V]", "axis no"=w343, "device handle"=w344) -> ("error out"=w340:T7)  [unwired: 2 in, 1 out]
            n169 = call <vilib>:"Add State(s) to Queue__JKI_lib_State_Machine.vi"("State(s) in (\"\")"=w347) -> ("States Out"=w346:string)  [unwired: 14 in]
          }
          event "axis 2:\nDCLevel [V]": Value Change {
            w351 = u8 1 items=["1", "2", "3", "4", "5", "6", "7", "8", "9"] ("axis no")
            n170 = event-data() -> ()  [unwired: 1 in, 6 out]
            n171 = Unbundle By Name(w353) -> ("handle"=w352:i32)
            n172 = call "ANC350_DCLevel.vi"("error in"=w350, "DCLevel [V]"="axis 2:\nDCLevel [V]", "axis no"=w351, "device handle"=w352) -> ("error out"=w349:T7)  [unwired: 2 in, 1 out]
            n173 = call <vilib>:"Add State(s) to Queue__JKI_lib_State_Machine.vi"("State(s) in (\"\")"=w355) -> ("States Out"=w354:string)  [unwired: 14 in]
          }
          event "axis 1:\nFrequency [Hz]": Value Change {
            w359 = u8 0 items=["1", "2", "3", "4", "5", "6", "7", "8", "9"] ("axis no")
            n174 = event-data() -> ()  [unwired: 1 in, 6 out]
            n175 = Unbundle By Name(w361) -> ("handle"=w360:i32)
            n176 = call "ANC350_Frequency.vi"("error in"=w357, "PositionerFrequency [Hz]"="axis 1:\nFrequency [Hz]", "axis no"=w359, "device handle"=w360) -> ("error out"=w356:T7)  [unwired: 2 in, 1 out]
            n177 = call <vilib>:"Add State(s) to Queue__JKI_lib_State_Machine.vi"("State(s) in (\"\")"=w363) -> ("States Out"=w362:string)  [unwired: 14 in]
          }
          event "axis 2:\nFrequency [Hz]": Value Change {
            w367 = u8 1 items=["1", "2", "3", "4", "5", "6", "7", "8", "9"] ("axis no")
            n178 = event-data() -> ()  [unwired: 1 in, 6 out]
            n179 = Unbundle By Name(w369) -> ("handle"=w368:i32)
            n180 = call "ANC350_Frequency.vi"("error in"=w366, "PositionerFrequency [Hz]"="axis 2:\nFrequency [Hz]", "axis no"=w367, "device handle"=w368) -> ("error out"=w365:T7)  [unwired: 2 in, 1 out]
            n181 = call <vilib>:"Add State(s) to Queue__JKI_lib_State_Machine.vi"("State(s) in (\"\")"=w371) -> ("States Out"=w370:string)  [unwired: 14 in]
          }
          event "axis 1:\ncap. measure": Value Change {
            w375 = u8 0 items=["1", "2", "3", "4", "5", "6", "7", "8", "9"] ("axis no")
            n182 = event-data() -> ()  [unwired: 1 in, 6 out]
            n183 = Unbundle By Name(w377) -> ("handle"=w376:i32)
            n184 = case shown="True" "axis 1:\ncap. measure" {
              tunnel: w376 -> [_ w385]
              tunnel: w375 -> [_ w384]
              tunnel: w374 -> [w380 w383]
              tunnel: [w380 w382] -> w373
              frame False {
              }
              frame True {
                n185 = call "ANC350_CapMeasure.vi"("error in"=w383, "axis no"=w384, "device handle"=w385) -> ("error out"=w382:T7, "Capacitance"=→"axis 1:\nCapacitance":i32)  [unwired: 2 in, 1 out]
              }
            }
            n186 = call <vilib>:"Add State(s) to Queue__JKI_lib_State_Machine.vi"("State(s) in (\"\")"=w379) -> ("States Out"=w378:string)  [unwired: 14 in]
          }
          event "axis 2:\ncap. measure": Value Change {
            w389 = u8 1 items=["1", "2", "3", "4", "5", "6", "7", "8", "9"] ("axis no")
            n187 = event-data() -> ()  [unwired: 1 in, 6 out]
            n188 = Unbundle By Name(w391) -> ("handle"=w390:i32)
            n189 = case shown="True" "axis 2:\ncap. measure" {
              tunnel: w390 -> [_ w399]
              tunnel: w389 -> [_ w398]
              tunnel: w388 -> [w394 w397]
              tunnel: [w394 w396] -> w387
              frame False {
              }
              frame True {
                n190 = call "ANC350_CapMeasure.vi"("error in"=w397, "axis no"=w398, "device handle"=w399) -> ("error out"=w396:T7, "Capacitance"=→"axis 2:\nCapacitance":i32)  [unwired: 2 in, 1 out]
              }
            }
            n191 = call <vilib>:"Add State(s) to Queue__JKI_lib_State_Machine.vi"("State(s) in (\"\")"=w393) -> ("States Out"=w392:string)  [unwired: 14 in]
          }
          event "axis 1:\ncontrol mode": Value Change {
            w403 = u8 0 items=["1", "2", "3", "4", "5", "6", "7", "8", "9"] ("axis no")
            n192 = event-data() -> ()  [unwired: 1 in, 6 out]
            n193 = Unbundle By Name(w405) -> ("handle"=w404:i32)
            n194 = call "ANC350_AmplitudeControl.vi"("error in"=w402, "control mode"="axis 1:\ncontrol mode", "axis no"=w403, "device handle"=w404) -> ("error out"=w401:T7)  [unwired: 2 in, 1 out]
            n195 = call <vilib>:"Add State(s) to Queue__JKI_lib_State_Machine.vi"("State(s) in (\"\")"=w407) -> ("States Out"=w406:string)  [unwired: 14 in]
          }
          event "axis 2:\ncontrol mode": Value Change {
            w411 = u8 1 items=["1", "2", "3", "4", "5", "6", "7", "8", "9"] ("axis no")
            n196 = event-data() -> ()  [unwired: 1 in, 6 out]
            n197 = Unbundle By Name(w413) -> ("handle"=w412:i32)
            n198 = call "ANC350_AmplitudeControl.vi"("error in"=w410, "control mode"="axis 2:\ncontrol mode", "axis no"=w411, "device handle"=w412) -> ("error out"=w409:T7)  [unwired: 2 in, 1 out]
            n199 = call <vilib>:"Add State(s) to Queue__JKI_lib_State_Machine.vi"("State(s) in (\"\")"=w415) -> ("States Out"=w414:string)  [unwired: 14 in]
          }
          event "axis 1:\nOutput": Value Change {
            w417 = u8 0 items=["1", "2", "3", "4", "5", "6", "7", "8", "9"] ("axis no")
            n200 = event-data() -> ()  [unwired: 1 in, 6 out]
            n201 = Unbundle By Name(w421) -> ("handle"=w420:i32)
            n202 = call "ANC350_SetOutput.vi"("error in"=w419, "enable"="axis 1:\nOutput", "axis no"=w417, "device handle"=w420) -> ("error out"=w418:T7)  [unwired: 2 in, 1 out]
            n203 = disable-structure shown="Disabled" {
              frame Disabled {
                n204 = Get Date/Time In Seconds() -> (seconds since 1Jan1904=w424:timestamp)
                n205 = local write "last move time"(w424) -> ()
              }
              frame Enabled {
              }
            }
            n206 = call <vilib>:"Add State(s) to Queue__JKI_lib_State_Machine.vi"("State(s) in (\"\")"=w423) -> ("States Out"=w422:string)  [unwired: 14 in]
          }
          event "axis 2:\nOutput": Value Change {
            w426 = u8 1 items=["1", "2", "3", "4", "5", "6", "7", "8", "9"] ("axis no")
            n207 = event-data() -> ()  [unwired: 1 in, 6 out]
            n208 = Unbundle By Name(w430) -> ("handle"=w429:i32)
            n209 = call "ANC350_SetOutput.vi"("error in"=w428, "enable"="axis 2:\nOutput", "axis no"=w426, "device handle"=w429) -> ("error out"=w427:T7)  [unwired: 2 in, 1 out]
            n210 = disable-structure shown="Disabled" {
              frame Disabled {
                n211 = Get Date/Time In Seconds() -> (seconds since 1Jan1904=w433:timestamp)
                n212 = local write "last move time"(w433) -> ()
              }
              frame Enabled {
              }
            }
            n213 = call <vilib>:"Add State(s) to Queue__JKI_lib_State_Machine.vi"("State(s) in (\"\")"=w432) -> ("States Out"=w431:string)  [unwired: 14 in]
          }
          event "axis 1:\nstop detection": Value Change {
            w437 = u8 0 items=["1", "2", "3", "4", "5", "6", "7", "8", "9"] ("axis no")
            n214 = event-data() -> ()  [unwired: 1 in, 6 out]
            n215 = Unbundle By Name(w439) -> ("handle"=w438:i32)
            n216 = call "ANC350_StopDetection.vi"("error in"=w436, "enable"="axis 1:\nstop detection", "axis no"=w437, "device handle"=w438) -> ("error out"=w435:T7)  [unwired: 2 in, 1 out]
            n217 = call <vilib>:"Add State(s) to Queue__JKI_lib_State_Machine.vi"("State(s) in (\"\")"=w441) -> ("States Out"=w440:string)  [unwired: 14 in]
          }
          event "axis 2:\nstop detection": Value Change {
            w445 = u8 1 items=["1", "2", "3", "4", "5", "6", "7", "8", "9"] ("axis no")
            n218 = event-data() -> ()  [unwired: 1 in, 6 out]
            n219 = Unbundle By Name(w447) -> ("handle"=w446:i32)
            n220 = call "ANC350_StopDetection.vi"("error in"=w444, "enable"="axis 2:\nstop detection", "axis no"=w445, "device handle"=w446) -> ("error out"=w443:T7)  [unwired: 2 in, 1 out]
            n221 = call <vilib>:"Add State(s) to Queue__JKI_lib_State_Machine.vi"("State(s) in (\"\")"=w449) -> ("States Out"=w448:string)  [unwired: 14 in]
          }
          event "axis 1:\nStop moving": Value Change {
            w453 = u8 0 items=["1", "2", "3", "4", "5", "6", "7", "8", "9"] ("axis no")
            n222 = event-data() -> ()  [unwired: 1 in, 6 out]
            n223 = Unbundle By Name(w455) -> ("handle"=w454:i32)
            n224 = case shown="False" "axis 1:\nStop moving" {
              tunnel: w454 -> [_ w462]
              tunnel: w453 -> [_ w461]
              tunnel: w452 -> [w458 w460]
              tunnel: [w458 w459] -> w451
              frame False {
              }
              frame True {
                n225 = call "ANC350_StopMoving.vi"("error in"=w460, "axis no"=w461, "device handle"=w462) -> ("error out"=w459:T7)  [unwired: 3 in, 1 out]
              }
            }
            n226 = call <vilib>:"Add State(s) to Queue__JKI_lib_State_Machine.vi"("State(s) in (\"\")"=w457) -> ("States Out"=w456:string)  [unwired: 14 in]
          }
          event "axis 2:\nStop moving": Value Change {
            w466 = u8 1 items=["1", "2", "3", "4", "5", "6", "7", "8", "9"] ("axis no")
            n227 = event-data() -> ()  [unwired: 1 in, 6 out]
            n228 = Unbundle By Name(w468) -> ("handle"=w467:i32)
            n229 = case shown="True" "axis 2:\nStop moving" {
              tunnel: w467 -> [_ w475]
              tunnel: w466 -> [_ w474]
              tunnel: w465 -> [w471 w473]
              tunnel: [w471 w472] -> w464
              frame False {
              }
              frame True {
                n230 = call "ANC350_StopMoving.vi"("error in"=w473, "axis no"=w474, "device handle"=w475) -> ("error out"=w472:T7)  [unwired: 3 in, 1 out]
              }
            }
            n231 = call <vilib>:"Add State(s) to Queue__JKI_lib_State_Machine.vi"("State(s) in (\"\")"=w470) -> ("States Out"=w469:string)  [unwired: 14 in]
          }
          event "both axes: Output": Value Change {
            n232 = event-data() -> ()  [unwired: 1 in, 6 out]
            n233 = disable-structure shown="Disabled" {
              frame Disabled {
                n234 = local write "axis 2:\nOutput"("both axes: Output") -> ()
                n235 = local write "axis 1:\nOutput"("both axes: Output") -> ()
                n236 = property on="axis 1:\nOutput" class="Bool (strict)"("Val(Sgnl)"="both axes: Output") -> ()  [unwired: 2 in, 2 out]
                n237 = property on="axis 2:\nOutput" class="Bool (strict)"("Val(Sgnl)"="both axes: Output") -> ()  [unwired: 2 in, 2 out]
              }
              frame Enabled {
              }
            }
            n238 = call <vilib>:"Add State(s) to Queue__JKI_lib_State_Machine.vi"("State(s) in (\"\")"=w479) -> ("States Out"=w478:string)  [unwired: 14 in]
          }
          event "static amplitude (mV)": Value Change {
            n239 = event-data() -> ()  [unwired: 1 in, 6 out]
            n240 = local read "set static amplitude\nwhen moving"() -> (w481:bool)
            n241 = local read "static amplitude (mV)"() -> (w482:dbl)
            n242 = Unbundle By Name(w486) -> ("handle"=w485:i32)
            n243 = case shown="False" w481 {
              tunnel: w485 -> [w492 _]
              tunnel: w484 -> [w491 w493]
              tunnel: [w490 w493] -> w483
              tunnel: w482 -> [w489 _]
              frame False {
                n244 = call "ANC350_StaticAmplitude.vi"("error in"=w491, "static amplitude"=w489, "device handle"=w492) -> ("error out"=w490:T7)  [unwired: 3 in, 1 out]
              }
              frame True {
              }
            }
            n245 = call <vilib>:"Add State(s) to Queue__JKI_lib_State_Machine.vi"("State(s) in (\"\")"=w488) -> ("States Out"=w487:string)  [unwired: 14 in]
          }
          event Panel Close? {
            # "Discard the event because we'll close the front panel ourselves in Macro: Exit"
            # "Close Panel button (pressed) Event\n(this executes Macro: Exit to terminate the VI)"
            n246 = event-data() -> ()  [unwired: 1 in, 1 out]
            n247 = call <vilib>:"Add State(s) to Queue__JKI_lib_State_Machine.vi"("State(s) in Front (\"\")"="Macro: Exit", "State(s) in (\"\")"=w499) -> ("States Out"=w498:string)  [unwired: 13 in]
            n248 = event-data("Discard?"=TRUE) -> ()  [unwired: 1 in, 1 out]
          }
        }
      }
      frame "---------- Core ----------" {
        # "Do not put any code in this frame.\n(it is a separator no-op)"
        n249 = call <vilib>:"Add State(s) to Queue__JKI_lib_State_Machine.vi"("State(s) in (\"\")"=w503) -> ("States Out"=w502:string)  [unwired: 14 in]
      }
      frame Default {
        w513 = 42 items=["No error", "Argument error", "Memory is full", "Out of zone", "End of file", "File already open", "Generic file I/O error", "File not found", "File permission error", "Disk is full", "Duplicate path", "Too many files open", "System feature not enabled", "Resource file not found", "Cannot add resource", "Resource not found", "Image not found", "Image memory error", "Pen does not exist", "Config type invalid", "Config token not found", "Config parse error", "Config memory error", "Bad external code format", "Bad external code offset", "External code not present", "Null window", "Destroy window error", "Null menu", "Print aborted", "Bad print record", "Print driver error", "Windows error during printing", "Memory error during printing", "Print dialog error", "Generic print error", "Invalid device refnum", "Device not found", "Device parameter error", "Device unit error", "Cannot open device", "Device call aborted", "Generic error", "Cancelled by user", "Object ID too low", "Object ID too high", "Object not in heap", "Unknown heap", "Unknown object (invalid DefProc)", "Unknown object (DefProc not in table)", "Message out of range", "Invalid (null) method", "Unknown message", "Manager call not supported", "Bad address", "Network operation in progress", "Network operation timed out", "Connection is busy", "Network attribute not supported", "Network error", "Address in use", "System out of memory", "Connection aborted", "Connection refused", "Not connected", "Already connected", "Connection closed", "Initialization error (interapplication manager)", "Bad occurrence", "Wait on unbound occurrence handler", "Occurrence queue overflow", "Datalog type conflict", "Unused", "Unrecognized type (interapplication manager)", "Memory corrupt", "Failed to make temporary DLL", "Old CIN version", "Drag socket not found", "Failed to load drop-object", "Failed to register OLE object", "Failed to release OLE object", "Format specifier type mismatch", "Unknown format specifier", "Too few format specifiers", "Too many format specifiers", "Scan failed", "Newer CIN version", "Error converting to variant", "Runtime menu error", "Password tampered", "Variant attribute not found", "Incompatible variant data type", "Event data is not available", "Event Store is not present", "Occurrence is not found", "Event Queue is not created", "Event info is not available", "Refnum passed is NULL", "Error retrieving Class GUID", "Error retrieving CoClass GUID", "Error retrieving TypeLib GUID.", "Bad built application magic bytes.", "Specific driver is different from the specific driver associated with the Logical Name.", "There is no session opened to the class driver.", "Max Error", "MAX - Error with config objects", "MAX - Error loading configuration", "MAX - Group not supported"]
        # "Current State"
        # "Do not delete, rename, or modify this frame.\n(this is used to capture unhandled states and typos)"
        # "Handle mistyped state name (developer tool)"
        n250 = Format Into String(format string="Software Exception: Unhandled State \"%s\"." ("message"), error in=w509, w504) -> (resulting string=w512:string, error out=w511:errorcluster)  [unwired: 1 in]
        n251 = call <vilib>:"Error Cluster From Error Code.vi"("show call chain? (False)"=TRUE, "error in (no error)"=w511, "error message (\"\")"=w512, "error code (0)"=w513) -> ("error out"=w510:errorcluster)  [unwired: 5 in]
        n252 = call <vilib>:"Add State(s) to Queue__JKI_lib_State_Machine.vi"("State(s) in (\"\")"=w508) -> ("States Out"=w507:string)  [unwired: 14 in]
      }
      frame "Initialize Core Data" {
        # "Do not delete, rename, or modify this frame.\n(this is used to determine panel behavior on exit)"
        # "originally closed?"
        # "exe?"
        # "If panel starts closed or is an EXE, then close it when we exit"
        n253 = property class="VI"() -> ("Front Panel.Open"=w522:bool)  [unwired: 2 in, 2 out]
        n254 = property class="App"() -> ("App.Kind"=w521:T2)  [unwired: 2 in, 2 out]
        n255 = control-ref of="Current VI Reference"() -> (w515:refnum<vi>)
        n256 = Not(x=w522) -> (.not. x?=w519:bool)
        n257 = Equal?(x=w521, y=T2."Run Time System" ("Application:Kind")) -> (x = y?=w518:bool)
        n258 = Or(x=w519, y=w518) -> (x .or. y?=w516:bool)
        n259 = Bundle By Name(cluster=w517, "Core.Current VI Reference"=w515, "Core.Close Panel on Exit?"=w516) -> (w524:T8)
        n260 = call <vilib>:"Add State(s) to Queue__JKI_lib_State_Machine.vi"("State(s) in (\"\")"=w526) -> ("States Out"=w525:string)  [unwired: 14 in]
      }
      frame "Error Handler" {
        # "Unhandled Error -- Display it"
        # "Handle any errors here.\nYou can also output any states to clean-up after errors occur"
        # "Clear error"
        n261 = call <vilib>:"General Error Handler.vi"("error in (no error)"=w528) -> ()  [unwired: 10 in, 5 out]
        n262 = call <vilib>:"Add State(s) to Queue__JKI_lib_State_Machine.vi"("State(s) in Front (\"\")"="/* Post Error States", "State(s) in (\"\")"=w532) -> ("States Out"=w531:string)  [unwired: 13 in]
      }
      frame "Exit" {
        # "Do not put any code in this frame.\n(No errors that occur here will be handled.)"
        n263 = call <vilib>:"Add State(s) to Queue__JKI_lib_State_Machine.vi"("State(s) in (\"\")"=w537) -> ("States Out"=w536:string)  [unwired: 14 in]
      }
      frame "---------- Data ----------" {
        # "Do not put any code in this frame.\n(It is a separator no-op. You can make a copy of this frame to create a new Data frame)"
        n264 = call <vilib>:"Add State(s) to Queue__JKI_lib_State_Machine.vi"("State(s) in (\"\")"=w541) -> ("States Out"=w540:string)  [unwired: 14 in]
      }
      frame "Data: Initialize" {
        w542 = 0  # handle
        w543 = T9 {"Current VI Reference"=refnum, "Close Panel on Exit?"=FALSE}  # Core
        # "do not delete - used by framework"
        # "Expand Bundle to add new data elements to shift register data."
        # "Data names and types of shift register data are defined by this bundle."
        # "Initialize the shift-register data, here.\n(data names are defined by what you wire into the bundle function)"
        n265 = Bundle("Core"=w543, "handle"=w542) -> (w545:T8)  [unwired: 1 in]
        n266 = call <vilib>:"Add State(s) to Queue__JKI_lib_State_Machine.vi"("State(s) in (\"\")"=w547) -> ("States Out"=w546:string)  [unwired: 14 in]
      }
      frame "Data: Cleanup" {
        # "Cleanup any data and references, here.\n(this is called automatically, by the Macro: Exit)"
        n267 = Unbundle By Name(w548) -> ("Core.Current VI Reference"=w551:refnum<vi>)
        n268 = Close Reference(reference=w551, error in (no error)=w550) -> (error out=w549:errorcluster)
        n269 = call <vilib>:"Add State(s) to Queue__JKI_lib_State_Machine.vi"("State(s) in (\"\")"=w553) -> ("States Out"=w552:string)  [unwired: 14 in]
      }
      frame "---------- UI ----------" {
        # "Do not put any code in this frame.\n(It is a separator no-op. You can make a copy of this frame to create a new UI frame)"
        n270 = call <vilib>:"Add State(s) to Queue__JKI_lib_State_Machine.vi"("State(s) in (\"\")"=w557) -> ("States Out"=w556:string)  [unwired: 14 in]
      }
      frame "UI: Initialize" {
        w558 = FALSE ("OK")
        w562 = FALSE ("axis 1:\nAbsolute")
        w563 = FALSE ("axis 1:\nAbsolute")
        w560 = FALSE ("axis 1:\nAbsolute")
        w564 = FALSE ("axis 1: \nTarget GND")
        # "initialize buttons and graphs....."
        # "Initialize the User Interface, here.\n(this is called automatically, by the Macro: Init)"
        n271 = local write "axis 1:\nSingle Circle Mode"(TRUE ("axis 1: \nTarget GND")) -> ()
        n272 = local write "axis 2:\nSingle Circle Mode"(FALSE ("axis 1:\nAbsolute")) -> ()
        n273 = local write "axis 1: \nTarget GND"(w564) -> ()
        n274 = local write "axis 2: \nTarget GND"(w564) -> ()
        n275 = local write "axis 2:\nAbsolute"(w560) -> ()
        n276 = local write "axis 1:\nAbsolute"(w560) -> ()
        n277 = local write "axis 1:\nRelative"(w560) -> ()
        n278 = local write "axis 2:\nRelative"(w560) -> ()
        n279 = local write "axis 2:\ncap. measure"(w562) -> ()
        n280 = local write "axis 1:\ncap. measure"(w562) -> ()
        n281 = local write "axis 2:\nOutput"(w560) -> ()
        n282 = local write "axis 1:\nOutput"(w560) -> ()
        n283 = local write "axis 1:\nsingle step fwd"(w563) -> ()
        n284 = local write "axis 2:\nsingle step fwd"(w563) -> ()
        n285 = local write "axis 1:\ncontinuous fwd"(w563) -> ()
        n286 = local write "axis 2:\ncontinuous fwd"(w563) -> ()
        n287 = local write "axis 1:\nsingle step back"(w563) -> ()
        n288 = local write "axis 2:\nsingle step back"(w563) -> ()
        n289 = local write "axis 1:\ncontinuous back"(w563) -> ()
        n290 = local write "axis 2:\ncontinuous back"(w563) -> ()
        n291 = local write "OK"(w558) -> ()
        n292 = local write "Remote mode"(w558) -> ()
        n293 = local write "both axes: Output"(w558) -> ()
        n294 = disable-structure shown="Disabled" {
          frame Disabled {
            w569 = 0.0 ("axis 1:\nAmplitude [V]")
            w570 = 0 ("axis 1:\nFrequency [Hz]")
            w571 = 0.0 ("axis 1:\nAmplitude [V]")
            w572 = 1000 ("axis 1:\nFrequency [Hz]")
            w573 = 30.0 ("axis 1:\nAmplitude [V]")
            n295 = local write "axis 1:\nAmplitude [V]"(w573) -> ()
            n296 = local write "axis 2:\nAmplitude [V]"(w573) -> ()
            n297 = local write "axis 1:\nFrequency [Hz]"(w572) -> ()
            n298 = local write "axis 2:\nFrequency [Hz]"(w572) -> ()
            n299 = local write "axis 1:\nDCLevel [V]"(w571) -> ()
            n300 = local write "axis 2:\nDCLevel [V]"(w571) -> ()
            n301 = local write "axis 1:\nsp rot count"(w570) -> ()
            n302 = local write "axis 2:\nsp rot count"(w570) -> ()
            n303 = local write "axis 1:\nsp position °"(w569) -> ()
            n304 = local write "axis 2:\nsp position °"(w569) -> ()
          }
          frame Enabled {
          }
        }
        n305 = call <vilib>:"Add State(s) to Queue__JKI_lib_State_Machine.vi"("State(s) in (\"\")"=w568) -> ("States Out"=w567:string)  [unwired: 14 in]
      }
      frame "UI: Cursor Set" {
        # "Argument"
        # "Set and Unset Cursor Busy.\n(Usage: \"UI: Cursor Set >> Busy|Idle\")"
        n306 = case shown="\"Idle\", Default" w574 {
          tunnel: w576 -> [w581 w583]
          tunnel: [w580 w582] -> w575
          frame "Idle", Default {
            n307 = call <vilib>:"Unset Busy.vi"("error in (no error)"=w581) -> ("error out"=w580:errorcluster)  [unwired: 10 in]
          }
          frame "Busy" {
            n308 = call <vilib>:"Set Busy.vi"("error in (no error)"=w583) -> ("error out"=w582:errorcluster)  [unwired: 9 in, 1 out]
          }
        }
        n309 = call <vilib>:"Add State(s) to Queue__JKI_lib_State_Machine.vi"("State(s) in (\"\")"=w579) -> ("States Out"=w578:string)  [unwired: 14 in]
      }
      frame "UI: Front Panel State" {
        # "Argument"
        # "Set Front Panel Open or Closed\n(Usage: \"UI: Front Panel State >> Open|Close\")"
        n310 = Unbundle By Name(w586) -> ("Core.Current VI Reference"=w585:refnum<vi>)
        n311 = case shown="\"Open\", Default" w584 {
          tunnel: w588 -> [w594 w607]
          tunnel: [w596 w608] -> w587
          tunnel: w585 -> [w595 w605]
          frame "Open", Default {
            n312 = property class="VI"(reference=w595, error in=w594) -> (reference out=w592:refnum<vi>, error out=w593:errorcluster, "Front Panel.Open"=w591:bool)
            n313 = case shown="False" w591 {
              tunnel: [w599 w602] -> w596
              tunnel: w593 -> [w598 w602]
              tunnel: w592 -> [w597 _]
              frame False {
                n314 = invoke class="VI" method="FP.Open"(reference=w597, error in=w598, "Activate"=TRUE, "State"=T3."Standard") -> (error out=w599:errorcluster)  [unwired: 1 in, 4 out]
              }
              frame True {
              }
            }
          }
          frame "Close" {
            n315 = property class="VI"(reference=w605, error in=w607) -> (reference out=w604:refnum<vi>, error out=w606:errorcluster, "Front Panel.Open"=w603:bool)
            n316 = case shown="True" w603 {
              tunnel: [w609 w612] -> w608
              tunnel: w606 -> [w609 w611]
              tunnel: w604 -> [_ w610]
              frame False {
              }
              frame True {
                n317 = invoke class="VI" method="FP.Close"(reference=w610, error in=w611) -> (error out=w612:errorcluster)  [unwired: 1 in, 2 out]
              }
            }
          }
        }
        n318 = call <vilib>:"Add State(s) to Queue__JKI_lib_State_Machine.vi"("State(s) in (\"\")"=w590) -> ("States Out"=w589:string)  [unwired: 14 in]
      }
      frame "---------- Macro ----------" {
        # "Do not put any code in this frame.\n(It is a separator no-op. You can make a copy of this frame to create a new Macro frame)"
        n319 = call <vilib>:"Add State(s) to Queue__JKI_lib_State_Machine.vi"("State(s) in (\"\")"=w616) -> ("States Out"=w615:string)  [unwired: 14 in]
      }
      frame "Macro: Initialize" {
        w617 = "Data: Initialize\nInitialize Core Data\nUI: Initialize\nUI: Front Panel State >> Open\nAttocube: Initialize"  # Data: Initialize Initialize Core Data UI: Initialize UI: Front Panel State >> Open Attocube: Initialize
        # "Initialization Macro\n(This is called once, when the VI starts)"
        n320 = call <vilib>:"Add State(s) to Queue__JKI_lib_State_Machine.vi"("State(s) in Front (\"\")"=w617, "State(s) in (\"\")"=w621) -> ("States Out"=w620:string)  [unwired: 13 in]
      }
      frame "Macro: Exit" {
        w625 = u8 1 items=["1", "2", "3", "4", "5", "6", "7", "8", "9"] ("axis no")
        w628 = u8 0 items=["1", "2", "3", "4", "5", "6", "7", "8", "9"] ("axis no")
        w632 = u8 1 items=["1", "2", "3", "4", "5", "6", "7", "8", "9"] ("axis no")
        w633 = u8 0 items=["1", "2", "3", "4", "5", "6", "7", "8", "9"] ("axis no")
        # "Exit Macro\n(This is called once, when the VI exits)"
        n321 = Unbundle By Name(w645) -> ("Core.Close Panel on Exit?"=w644:bool, "handle"=w637:i32)
        n322 = call "ANC350_StopMoving.vi"("error in"=w635, "axis no"=w633, "device handle"=w637) -> ("error out"=w634:T7, "device handle Out"=w636:i32)  [unwired: 3 in]
        n323 = call "ANC350_StopMoving.vi"("error in"=w634, "axis no"=w632, "device handle"=w636) -> ("error out"=w629:T7, "device handle Out"=w631:i32)  [unwired: 3 in]
        n324 = call "ANC350_SetOutput.vi"("error in"=w629, "enable"=FALSE, "axis no"=w628, "device handle"=w631) -> ("error out"=w624:T7, "device handle out"=w627:i32)  [unwired: 2 in]
        n325 = Select(t="UI: Front Panel State >> Close", s=w644, f="") -> (s? t:f=w641:string)
        n326 = call "ANC350_SetOutput.vi"("error in"=w624, "enable"=FALSE, "axis no"=w625, "device handle"=w627) -> ("error out"=w622:T7, "device handle out"=w623:i32)  [unwired: 2 in]
        n327 = call <vilib>:"Add State(s) to Queue__JKI_lib_State_Machine.vi"("State(s) in (\"\")"=w641, "State(s) at Back (\"\")"="Data: Cleanup\nExit") -> ("States Out"=w639:string)  [unwired: 13 in]
        n328 = call "ANC350_Close.vi"("error in"=w622, "device handle"=w623) -> ("error out"=w638:T7)  [unwired: 5 in]
        n329 = call <vilib>:"Add State(s) to Queue__JKI_lib_State_Machine.vi"("State(s) in Front (\"\")"=w639, "State(s) in (\"\")"=w647) -> ("States Out"=w646:string)  [unwired: 13 in]
      }
      frame "---------- New Category ----------" {
        # "Template Separator\n(You can make a copy of, or modify, this frame)"
        n330 = call <vilib>:"Add State(s) to Queue__JKI_lib_State_Machine.vi"("State(s) in (\"\")"=w651) -> ("States Out"=w650:string)  [unwired: 14 in]
      }
      frame "Attocube: Initialize" {
        w655 = u8 1 items=["1", "2", "3", "4", "5", "6", "7", "8", "9"] ("axis no")
        w658 = u8 0 items=["1", "2", "3", "4", "5", "6", "7", "8", "9"] ("axis no")
        n331 = disable-structure shown="Disabled" {
          frame Disabled {
            n332 = Get Date/Time In Seconds() -> (seconds since 1Jan1904=w667:timestamp)
            n333 = local write "last move time"(w667) -> ()
          }
          frame Enabled {
          }
        }
        n334 = flat-sequence {
          tunnel: [w668] -> w661
          tunnel: [w669] -> w660
          tunnel: [w668] -> w659
          frame #0 {
            n335 = call "ANC350_Check.vi"() -> ()  [unwired: 6 in, 2 out]
          }
          frame #1 {
            n336 = call "ANC350_Connect.vi"("device no"=0) -> ("error out"=w669:T7, "handle"=w668:i32)  [unwired: 5 in]
            "handle" <- w668
          }
        }
        n337 = Bundle By Name(cluster=w664, "handle"=w661) -> (w663:T8)
        n338 = call "ANC350_GetPosition.vi"("error in"=w660, "axis no"=w658, "device handle"=w659) -> ("error out"=w654:T7, 1:w657, "device handle Out"=w656:i32)  [unwired: 1 in, 1 out]
        n339 = local write "axis 1:\nsp position °"(w657) -> ()
        n340 = call "ANC350_GetPosition.vi"("error in"=w654, "axis no"=w655, "device handle"=w656) -> ("error out"=w653:T7, 1:w652)  [unwired: 1 in, 2 out]
        n341 = local write "axis 2:\nsp position °"(w652) -> ()
        n342 = call <vilib>:"Add State(s) to Queue__JKI_lib_State_Machine.vi"("State(s) in (\"\")"=w666, "State(s) at Back (\"\")"="Attocube: Query\nAttocube: Log to DSC\nAttocube: FGV" ("State(s) at Back (\"\")")) -> ("States Out"=w665:string)  [unwired: 13 in]
      }
      frame "Attocube: Query" {
        w710 = u8 0 items=["1", "2", "3", "4", "5", "6", "7", "8", "9"] ("axis no")
        w717 = u8 1 items=["1", "2", "3", "4", "5", "6", "7", "8", "9"] ("axis no")
        w697 = u8 1 items=["1", "2", "3", "4", "5", "6", "7", "8", "9"] ("axis no")
        w718 = u8 0 items=["1", "2", "3", "4", "5", "6", "7", "8", "9"] ("axis no")
        w730 = u8 1 items=["1", "2", "3", "4", "5", "6", "7", "8", "9"] ("axis no")
        w732 = u8 0 items=["1", "2", "3", "4", "5", "6", "7", "8", "9"] ("axis no")
        n343 = Unbundle By Name(w734) -> ("handle"=w731:i32)
        n344 = local read "static amplitude (mV)"() -> (w672:dbl)
        n345 = local read "set static amplitude\nwhen moving"() -> (w674:bool)
        n346 = call "ANC350_GetRotCount.vi"("error in"=w733, "axis no"=w732, "device handle"=w731) -> ("error out"=w709:T7, "count"=→"axis 1:\nrot. count":i32, "device handle"=w711:i32)  [unwired: 2 in]
        n347 = call "ANC350_GetStatus.vi"("error in"=w709, "axis no"=w710, "device handle"=w711) -> ("error out"=w704:T7, "positioner status"=w702:T1, "axis no out"=w706:u8, "device handle Out"=w708:i32)  [unwired: 2 in, 3 out]
        "axis 1:\npositioner status" <- w702
        n348 = Less Or Equal?(x=w672, y=500.0) -> (x <= y?=w671:bool)
        n349 = Unbundle By Name(w702) -> ("moving"=w678:bool)
        n350 = local read "axis 2:\nCurrent position (°)"() -> (w686:dbl)
        n351 = local read "axis 1:\nCurrent position (°)"() -> (w701:dbl)
        n352 = Not(x=w678) -> (.not. x?=w675:bool)
        n353 = call "ANC350_GetPosition.vi"("error in"=w704, "axis no"=w706, "device handle"=w708) -> ("error out"=w703:T7, 1:w700, "position [µm/°/m°]"=w705:dbl, "device handle Out"=w707:i32)  [unwired: 1 in]
        n354 = And(x=w675, y=w674) -> (x .and. y?=w681:bool)
        n355 = Select(t=w701, s=w671, f=w700) -> (s? t:f=→"axis 1:\nCurrent position (°)" →"axis 1:\nCurrent position [µm/°/m°] 2":dbl)
        n356 = call "ANC350_GetSpeed.vi"("error in"=w703, "axis no"=w705, "device handle"=w707) -> ("error out"=w728:T7, "speed"=w722:i32, "device handle"=w729:i32)  [unwired: 2 in]
        n357 = call "ANC350_GetStepWidth.vi"("error in"=w728, "axis no"=w718, "device handle"=w729) -> ("error out"=w727:T7, "StepWidth"=→"axis 1:\nStepWidth":i32, "device handle"=w726:i32)  [unwired: 2 in]
        n358 = call "ANC350_GetRotCount.vi"("error in"=w727, "axis no"=w730, "device handle"=w726) -> ("error out"=w696:T7, "count"=→"axis 2:\nrot. count":i32, "device handle"=w698:i32)  [unwired: 2 in]
        n359 = call "ANC350_GetStatus.vi"("error in"=w696, "axis no"=w697, "device handle"=w698) -> ("error out"=w693:T7, "positioner status"=w689:T1, "axis no out"=w694:u8, "device handle Out"=w695:i32)  [unwired: 2 in, 3 out]
        "axis 2:\npositioner status" <- w689
        n360 = Unbundle By Name(w689) -> ("moving"=w677:bool)
        n361 = call "ANC350_GetPosition.vi"("error in"=w693, "axis no"=w694, "device handle"=w695) -> ("error out"=w692:T7, 1:w687, "position [µm/°/m°]"=w690:dbl, "device handle Out"=w691:i32)  [unwired: 1 in]
        n362 = Not(x=w677) -> (.not. x?=w688:bool)
        n363 = call "ANC350_GetSpeed.vi"("error in"=w692, "axis no"=w690, "device handle"=w691) -> ("error out"=w724:T7, "speed"=w713:i32, "device handle"=w725:i32)  [unwired: 2 in]
        n364 = And(x=w688, y=w674) -> (x .and. y?=w680:bool)
        n365 = Select(t=w686, s=w671, f=w687) -> (s? t:f=→"axis 2:\nCurrent position (°)" →"axis 2:\nCurrent position [µm/°/m°] 2":dbl)
        n366 = call "ANC350_GetStepWidth.vi"("error in"=w724, "axis no"=w717, "device handle"=w725) -> ("error out"=w684:T7, "StepWidth"=→"axis 2:\nStepWidth":i32, "device handle"=w682:i32)  [unwired: 2 in]
        n367 = Divide(x=w713, y=1000) -> (x/y=→"axis 2:\nspeed (°/s)":dbl)
        n368 = Divide(x=w722, y=1000) -> (x/y=→"axis 1:\nspeed (°/s)":dbl)
        n369 = And(x=w681, y=w680) -> (x .and. y?=w679:bool)
        n370 = Or(x=w678, y=w677) -> (x .or. y?=w676:bool)
        n371 = case shown="True" w679 {
          tunnel: w684 -> [w744 w748]
          tunnel: [w744 w747] -> w683
          tunnel: w682 -> [_ w746]
          frame False {
          }
          frame True {
            w745 = 1 ("static amplitude")
            n372 = local write "static amplitude (mV)"(w745) -> ()
            n373 = call "ANC350_StaticAmplitude.vi"("error in"=w748, "static amplitude"=w745, "device handle"=w746) -> ("error out"=w747:T7)  [unwired: 3 in, 1 out]
          }
        }
        n374 = case shown="False" w676 {
          frame False {
            # "output timeout"
            n375 = local read "last move time"() -> (w740:timestamp)
            n376 = Get Date/Time In Seconds() -> (seconds since 1Jan1904=w741:timestamp)
            n377 = Subtract(x=w741, y=w740) -> (x-y=w739:dbl)
            n378 = Greater?(x=w739, y=1800.0) -> (0:w737:bool)
            n379 = case shown="True" w737 {
              frame False {
              }
              frame True {
                n380 = disable-structure shown="Disabled" {
                  frame Disabled {
                    n381 = property on="both axes: Output" class="Bool (strict)"("Val(Sgnl)"=FALSE ("Value (Signaling)")) -> ()  [unwired: 2 in, 2 out]
                  }
                  frame Enabled {
                  }
                }
              }
            }
          }
          frame True {
            n382 = Get Date/Time In Seconds() -> (seconds since 1Jan1904=w743:timestamp)
            n383 = local write "last move time"(w743) -> ()
          }
        }
        n384 = call <vilib>:"Add State(s) to Queue__JKI_lib_State_Machine.vi"("State(s) in (\"\")"=w736) -> ("States Out"=w735:string)  [unwired: 14 in]
      }
      frame "Attocube: Log to DSC" {
        n385 = local read "axis 1:\nCurrent position (°)"() -> (w762:dbl)
        n386 = local read "axis 1:\npositioner status"() -> (w754:T1)
        n387 = local read "axis 1:\nFrequency [Hz]"() -> (w792:i32)
        n388 = local read "axis 1:\nAmplitude [V]"() -> (w752:dbl)
        n389 = local read "axis 1:\ncontrol mode"() -> (w791:enum16{"speed", "amplitude", "step size"})
        n390 = local read "axis 1:\nCapacitance"() -> (w794:i32)
        n391 = local read "axis 1:\nsp position °"() -> (w790:dbl)
        n392 = local read "axis 1:\nsp rot count"() -> (w789:i32)
        n393 = local read "axis 1:\nDCLevel [V]"() -> (w793:dbl)
        n394 = local read "axis 1:\nspeed (°/s)"() -> (w756:i32)
        n395 = local read "axis 1:\nStepWidth"() -> (w758:i32)
        n396 = local read "axis 1:\nrot. count"() -> (w760:i32)
        n397 = local read "axis 1:\nSingle Circle Mode"() -> (w778:bool)
        n398 = local read "axis 1:\nstop detection"() -> (w773:bool)
        n399 = Unbundle By Name(w754) -> ("moving"=w777:bool, "stop detected"=w776:bool, "sensor error"=w775:bool, "sensor disconnected"=w774:bool)
        n400 = local read "axis 1: \nTarget GND"() -> (w780:bool)
        n401 = local read "axis 1:\nOutput"() -> (w779:bool)
        n402 = Build Array(w752, w794, w762, w793, w792, w758, w791, w760, w790, w789, w756) -> (w782:dbl[])
        n403 = local read "axis 2:\nCurrent position (°)"() -> (w761:dbl)
        n404 = local read "static amplitude (mV)"() -> (w749:dbl)
        n405 = local read "axis 2:\nFrequency [Hz]"() -> (w786:i32)
        n406 = local read "axis 2:\nAmplitude [V]"() -> (w751:dbl)
        n407 = local read "axis 2:\ncontrol mode"() -> (w785:enum16{"speed", "amplitude", "step size"})
        n408 = local read "axis 2:\nsp position °"() -> (w784:dbl)
        n409 = local read "axis 2:\nCapacitance"() -> (w788:i32)
        n410 = local read "axis 2:\nsp rot count"() -> (w783:i32)
        n411 = local read "axis 2:\nDCLevel [V]"() -> (w787:dbl)
        n412 = local read "axis 2:\nspeed (°/s)"() -> (w755:i32)
        n413 = local read "axis 2:\nStepWidth"() -> (w757:i32)
        n414 = local read "axis 2:\nrot. count"() -> (w759:i32)
        n415 = Build Array(w780, w779, w778, w777, w776, w775, w774, w773) -> (w772:bool[])
        n416 = local read "axis 2:\npositioner status"() -> (w753:T1)
        n417 = Build Array (concatenate)(w782, w751, w788, w761, w787, w786, w757, w785, w759, w784, w783, w755, w749) -> (w781:dbl[])
        n418 = local read "axis 2:\nSingle Circle Mode"() -> (w769:bool)
        n419 = local read "axis 2:\nstop detection"() -> (w764:bool)
        n420 = Unbundle By Name(w753) -> ("moving"=w768:bool, "stop detected"=w767:bool, "sensor error"=w766:bool, "sensor disconnected"=w765:bool)
        n421 = local read "axis 2: \nTarget GND"() -> (w771:bool)
        n422 = local read "axis 2:\nOutput"() -> (w770:bool)
        n423 = Build Array (concatenate)(w772, w771, w770, w769, w768, w767, w766, w765, w764) -> (w763:bool[])
        n424 = call <vilib>:"Add State(s) to Queue__JKI_lib_State_Machine.vi"("State(s) in (\"\")"=w797) -> ("States Out"=w796:string)  [unwired: 14 in]
        n425 = call "Attocube_to_DSC.vi"("boolean"=w763, "dbl"=w781) -> ()  [unwired: 6 in]
      }
      frame "Attocube: FGV" {
        n426 = local read "axis 1:\nStop moving"() -> (w846:bool)
        n427 = local read "axis 2:\nStop moving"() -> (w847:bool)
        n428 = local read "set static amplitude\nwhen moving"() -> (w820:bool)
        n429 = local read "axis 1:\nAbsolute"() -> (w844:bool)
        n430 = local read "axis 2:\nAbsolute"() -> (w845:bool)
        n431 = local read "axis 1:\nOutput"() -> (w822:bool)
        n432 = local read "axis 2:\nOutput"() -> (w821:bool)
        n433 = local read "axis 1:\nFrequency [Hz]"() -> (w838:i32)
        n434 = local read "axis 1:\nFrequency [Hz]"() -> (w839:i32)
        n435 = local read "axis 1:\nAmplitude [V]"() -> (w834:dbl)
        n436 = local read "axis 2:\nAmplitude [V]"() -> (w835:dbl)
        n437 = local read "axis 1:\nsp position °"() -> (w840:dbl)
        n438 = local read "axis 2:\nsp position °"() -> (w841:dbl)
        n439 = local read "axis 1:\nsp rot count"() -> (w842:i32)
        n440 = local read "axis 2:\nsp rot count"() -> (w843:i32)
        n441 = local read "axis 1:\nDCLevel [V]"() -> (w836:dbl)
        n442 = local read "axis 2:\nDCLevel [V]"() -> (w837:dbl)
        n443 = Bundle By Name(cluster=T4 {"axis 1: Absolute"=FALSE, "axis 2: Absolute"=FALSE, "axis 1: Stop moving"=FALSE, "axis 2: Stop moving"=FALSE, "axis 1: Output"=FALSE, "axis 2: Output"=FALSE, "set static amplitude\nwhen moving"=TRUE} ("Actions OUT"), "axis 1: Absolute"=w844, "axis 2: Absolute"=w845, "axis 1: Stop moving"=w846, "axis 2: Stop moving"=w847, "axis 1: Output"=w822, "axis 2: Output"=w821, "set static amplitude\nwhen moving"=w820) -> (w811:T4)
        n444 = call "FGV - Attocube Actions.vi"("error in"=w815, "Function"=enum16{"write", "read"}."read") -> ("error out"=w814:errorcluster, "Actions OUT"=w812:T4)  [unwired: 4 in]
        n445 = Bundle By Name(cluster=T6 {"axis 1: Amplitude [V]"=40.0, "axis 2: Amplitude [V]"=35.0, "axis 1: DCLevel [V]"=0.0, "axis 2: DCLevel [V]"=0.0, "axis 1: Frequency [Hz]"=2500.0, "axis 2: Frequency [Hz]"=2500.0, "axis 1: sp position °"=107.0, "axis 2: sp position °"=78.5, "axis 1: sp rot count"=0.0, "axis 2: sp rot count"=0.0} ("Targets Out"), "axis 1: Amplitude [V]"=w834, "axis 2: Amplitude [V]"=w835, "axis 1: DCLevel [V]"=w836, "axis 2: DCLevel [V]"=w837, "axis 1: Frequency [Hz]"=w838, "axis 2: Frequency [Hz]"=w839, "axis 1: sp position °"=w840, "axis 2: sp position °"=w841, "axis 1: sp rot count"=w842, "axis 2: sp rot count"=w843) -> (w808:T6)
        n446 = Equal?(x=w811, y=w812) -> (x = y?=w806:bool)
        n447 = case shown="False" w806 {
          tunnel: [w863 w865] -> w810
          tunnel: w814 -> [w862 w865]
          tunnel: w811 -> [w861 _]
          frame False {
            n448 = call "FGV - Attocube Actions.vi"("error in"=w862, "Function"=enum16{"write", "read"}."write", "Actions IN"=w861) -> ("error out"=w863:errorcluster)  [unwired: 3 in, 1 out]
          }
          frame True {
          }
        }
        n449 = call "FGV - Attocube Targets.vi"("error in"=w810, "Function"=enum16{"write", "read"}."read") -> ("error out"=w807:errorcluster, "Targets Out"=w809:T6)  [unwired: 4 in]
        n450 = Equal?(x=w808, y=w809) -> (x = y?=w805:bool)
        n451 = case shown="False" w805 {
          tunnel: [w858 w860] -> w804
          tunnel: w808 -> [w857 _]
          tunnel: w807 -> [w856 w860]
          frame False {
            n452 = call "FGV - Attocube Targets.vi"("error in"=w856, "Function"=enum16{"write", "read"}."write", "Targets In"=w857) -> ("error out"=w858:errorcluster)  [unwired: 3 in, 1 out]
          }
          frame True {
          }
        }
        n453 = local read "axis 1:\nCurrent position (°)"() -> (w824:dbl)
        n454 = local read "axis 2:\nCurrent position (°)"() -> (w825:dbl)
        n455 = local read "axis 1:\npositioner status"() -> (w832:T1)
        n456 = local read "axis 2:\npositioner status"() -> (w833:T1)
        n457 = local read "axis 1:\nspeed (°/s)"() -> (w830:i32)
        n458 = local read "axis 2:\nspeed (°/s)"() -> (w831:i32)
        n459 = local read "axis 1:\nStepWidth"() -> (w828:i32)
        n460 = local read "axis 2:\nStepWidth"() -> (w829:i32)
        n461 = local read "axis 1:\nrot. count"() -> (w826:i32)
        n462 = local read "axis 2:\nrot. count"() -> (w827:i32)
        n463 = Bundle By Name(cluster=T5 {"axis 1: Current position (°)"=0.0, "axis 2: Current position (°)"=0.0, "axis 1: rot. count"=0.0, "axis 2: rot. count"=0.0, "axis 1: StepWidth"=0.0, "axis 2: StepWidth"=0.0, "axis 1: speed (°/s)"=0.0, "axis 2: speed (°/s)"=0.0, "axis 1: positioner status"={"moving"=FALSE, "stop detected"=FALSE, "sensor error"=FALSE, "sensor disconnected"=FALSE}, "axis 2: positioner status"={"moving"=FALSE, "stop detected"=FALSE, "sensor error"=FALSE, "sensor disconnected"=FALSE}} ("Status OUT"), "axis 1: Current position (°)"=w824, "axis 2: Current position (°)"=w825, "axis 1: rot. count"=w826, "axis 2: rot. count"=w827, "axis 1: StepWidth"=w828, "axis 2: StepWidth"=w829, "axis 1: speed (°/s)"=w830, "axis 2: speed (°/s)"=w831, "axis 1: positioner status"=w832, "axis 2: positioner status"=w833) -> (w802:T5)
        n464 = Wait (ms)(milliseconds to wait=u32 2000) -> ()  [unwired: 1 out]
        n465 = call "FGV - Attocube Status.vi"("error in"=w804, "Function"=enum16{"write", "read"}."read") -> ("error out"=w799:errorcluster, "Status OUT"=w801:T5)  [unwired: 4 in]
        n466 = Equal?(x=w802, y=w801) -> (x = y?=w800:bool)
        n467 = case shown="False" w800 {
          tunnel: [w853 w855] -> w823
          tunnel: w802 -> [w852 _]
          tunnel: w799 -> [w851 w855]
          frame False {
            n468 = call "FGV - Attocube Status.vi"("error in"=w851, "Function"=enum16{"write", "read"}."write", "Status IN"=w852) -> ("error out"=w853:errorcluster)  [unwired: 3 in, 1 out]
          }
          frame True {
          }
        }
        n469 = call <vilib>:"Add State(s) to Queue__JKI_lib_State_Machine.vi"("State(s) in (\"\")"=w850) -> ("States Out"=w849:string)  [unwired: 14 in]
      }
    }
  }
  n470 = disable-structure shown="Disabled" {
    frame Disabled {
      n471 = call "ANC350_StaticAmplitude.vi"() -> ()  [unwired: 6 in, 2 out]
    }
    frame Enabled {
    }
  }
  n472 = disable-structure shown="Disabled" {
    disable-tunnel: [w867 _] -> _
    disable-tunnel: [w866 _] -> _
    frame Disabled {
      n473 = call "visualize.vi"() -> ("small angle"=w866:sgl, "large axis angle"=w867:sgl)  [unwired: 9 in, 1 out]
    }
    frame Enabled {
    }
  }
